vi "CAEN SY5527.vi"() -> ()   [LabVIEW 2018]
uses:
  <vilib>/Instr/_visa.llb/VISA Configure Serial Port (Instr).vi
  <vilib>/Analysis/Matrix/Numeric/Conversions/Matrix To Array - RM.vi
  <vilib>/Analysis/Matrix/NI_Matrix.lvlib
  <instrlib>/CAENHVWrapper/CAENHVWrapper.lvlib
panel:
  in  "MEasuring":T1(tab)
  in  "logs_directory_path":path=path "C:/Users/NEOVP/Documents/HV_DATA"
  in  "Tempt-Presure-on-off":bool=TRUE
  in  "Group 2 log name":string="G2"
  in  "Offsets 2":bool
  out "Temperature [C]":dbl
  in  "COM Port":refnum<visa-resource-name>="COM5"
  out "Presure [Pa]":i32
  in  "Delay [s]":dbl=1.0
  in  "Graphs bachground Color":u32(colorbox)=16448250
  in  "IP Address":string="192.168.0.1"
  in  "Username":string="admin"
  in  "Password":string="admin"
  out "crate_map":string[][](table)
  in  "stop":bool
  in  "Group 1 log name":string="G1"
  in  "Offsets":bool
  in  "Pages Colors":u32[](array[colorbox])=[6901059, 10986955, 11240591, 32639, 32639, 32639, 32639, 16777224, 9868950, 4417895, 8686180, 8686180, 8686180, 8686180]
  in  "Group 1":u16(ring)=5 items=["B0--B1", "B0--B2", "B0--B3", "B1--B0", "B1--B2", "B1--B3", "B2--B0", "B2--B1", "B2--B3", "B3--B0", "B3--B1", "B3--B2"]
  in  "Group 2":u16(ring)=1 items=["B0--B1", "B0--B2", "B0--B3", "B1--B0", "B1--B2", "B1--B3", "B2--B0", "B2--B1", "B2--B3", "B3--B0", "B3--B1", "B3--B2"]
  in  "Set configure":bool
  out "S6-2L R_G1":dbl format="%.1e"
  out "S6-2R R_G1":dbl format="%.1e"
  out "S7-2L R_G1":dbl format="%.1e"
  out "S7-2R R_G1":dbl format="%.1e"
  out "S8-2L R_G1":dbl format="%.1e"
  out "S8-2R R_G1":dbl format="%.1e"
  out "E6-2L R_G1":dbl format="%.1e"
  out "E6-2R R_G1":dbl format="%.1e"
  out "E7-2L R_G1":dbl format="%.1e"
  out "E7-2R R_G1":dbl format="%.1e"
  out "E8-2L R_G1":dbl format="%.1e"
  out "E8-2R R_G1":dbl format="%.1e"
  out "E6-1L R_G1":dbl format="%.1e"
  out "E6-1R R_G1":dbl format="%.1e"
  out "E7-1L R_G1":dbl format="%.1e"
  out "E7-1R R_G1":dbl format="%.1e"
  out "E8-1L R_G1":dbl format="%.1e"
  out "E8-1R R_G1":dbl format="%.1e"
  out "S6-1L R_G1":dbl format="%.1e"
  out "S6-1R R_G1":dbl format="%.1e"
  out "S7-1L R_G1":dbl format="%.1e"
  out "S7-1R R_G1":dbl format="%.1e"
  out "S8-1L R_G1":dbl format="%.1e"
  out "S8-1R R_G1":dbl format="%.1e"
  out "E8-2R I":dbl format="%.3f"
  out "E8-2R V":dbl format="%.1f"
  out "8-R_Gr_L3":bool
  in  "Limits":cluster{dbl, dbl}(slide)={80.16806722689076, 30.252100840336134} scale=0.0..120.0
  out "E6-1R I":dbl format="%.3f"
  out "E6-1R V":dbl format="%.1f"
  out "E6-1L V":dbl format="%.1f"
  out "E6-1L I":dbl format="%.3f"
  out "E7-1R I":dbl format="%.3f"
  out "E7-1R V":dbl format="%.1f"
  out "E7-1L V":dbl format="%.1f"
  out "E7-1L I":dbl format="%.3f"
  out "E8-1R I":dbl format="%.3f"
  out "E8-1R V":dbl format="%.1f"
  out "E8-1L V":dbl format="%.1f"
  out "E8-1L I":dbl format="%.3f"
  out "E6-2R I":dbl format="%.3f"
  out "E6-2R V":dbl format="%.1f"
  out "E6-2L V":dbl format="%.1f"
  out "E6-2L I":dbl format="%.3f"
  out "E7-2R I":dbl format="%.3f"
  out "E7-2R V":dbl format="%.1f"
  out "E7-2L V":dbl format="%.1f"
  out "E7-2L I":dbl format="%.3f"
  out "E8-2L V":dbl format="%.1f"
  out "E8-2L I":dbl format="%.3f"
  out "S6-1R I":dbl format="%.3f"
  out "S6-1R V":dbl format="%.1f"
  out "S6-1L V":dbl format="%.1f"
  out "S6-1L I":dbl format="%.3f"
  out "S7-1R I":dbl format="%.3f"
  out "S7-1R V":dbl format="%.1f"
  out "S7-1L V":dbl format="%.1f"
  out "S7-1L I":dbl format="%.3f"
  out "S8-1R I":dbl format="%.3f"
  out "S8-1R V":dbl format="%.1f"
  out "S8-1L V":dbl format="%.1f"
  out "S8-1L I":dbl format="%.3f"
  out "S6-2R I":dbl format="%.3f"
  out "S6-2R V":dbl format="%.1f"
  out "S6-2L V":dbl format="%.1f"
  out "S6-2L I":dbl format="%.3f"
  out "S7-2R I":dbl format="%.3f"
  out "S7-2R V":dbl format="%.1f"
  out "S7-2L V":dbl format="%.1f"
  out "S7-2L I":dbl format="%.3f"
  out "S8-2R I":dbl format="%.3f"
  out "S8-2R V":dbl format="%.1f"
  out "S8-2L V":dbl format="%.1f"
  out "S8-2L I":dbl format="%.3f"
  out "6-L_Gr_L4":bool
  out "6-R_Gr_L4":bool
  out "7-L_Gr_L4":bool
  out "7-R_Gr_L4":bool
  out "8-L_Gr_L4":bool
  out "8-R_Gr_L4":bool
  out "6-L_Gr_L3":bool
  out "6-R_Gr_L3":bool
  out "7-L_Gr_L3":bool
  out "7-R_Gr_L3":bool
  out "8-L_Gr_L3":bool
  out "6-L_Gr_L2":bool
  out "6-R_Gr_L2":bool
  out "7-L_Gr_L2":bool
  out "7-R_Gr_L2":bool
  out "8-L_Gr_L2":bool
  out "8-R_Gr_L2":bool
  out "6-L_Gr_L1":bool
  out "6-R_Gr_L1":bool
  out "7-L_Gr_L1":bool
  out "7-R_Gr_L1":bool
  out "8-L_Gr_L1":bool
  out "8-R_Gr_L1":bool
  out "8-R_G_L1":bool
  out "8-L_G_L1":bool
  out "8-L_Y_L1":bool
  out "8-R_Y_L1":bool
  out "8-L_R_L1":bool
  out "6-R_R_L1":bool
  out "6-R_Y_L1":bool
  out "6-R_G_L1":bool
  out "6-L_R_L1":bool
  out "6-L_Y_L1":bool
  out "6-L_G_L1":bool
  out "7-R_G_L1":bool
  out "8-R_R_L1":bool
  out "7-L_R_L1":bool
  out "7-L_G_L1":bool
  out "7-R_R_L1":bool
  out "7-L_Y_L1":bool
  out "7-R_Y_L1":bool
  out "8-R_G_L3":bool
  out "8-L_G_L3":bool
  out "8-L_Y_L3":bool
  out "8-R_Y_L3":bool
  out "8-L_R_L3":bool
  out "6-R_R_L3":bool
  out "6-R_Y_L3":bool
  out "6-R_G_L3":bool
  out "6-L_R_L3":bool
  out "6-L_Y_L3":bool
  out "6-L_G_L3":bool
  out "7-R_G_L3":bool
  out "8-R_R_L3":bool
  out "7-L_R_L3":bool
  out "7-L_G_L3":bool
  out "7-R_R_L3":bool
  out "7-L_Y_L3":bool
  out "7-R_Y_L3":bool
  out "8-R_G_L2":bool
  out "8-L_G_L2":bool
  out "8-L_Y_L2":bool
  out "8-R_Y_L2":bool
  out "8-L_R_L2":bool
  out "6-R_R_L2":bool
  out "6-R_Y_L2":bool
  out "6-R_G_L2":bool
  out "6-L_R_L2":bool
  out "6-L_Y_L2":bool
  out "6-L_G_L2":bool
  out "7-R_G_L2":bool
  out "8-R_R_L2":bool
  out "7-L_R_L2":bool
  out "7-L_G_L2":bool
  out "7-R_R_L2":bool
  out "7-L_Y_L2":bool
  out "7-R_Y_L2":bool
  out "8-R_G_L4":bool
  out "8-L_G_L4":bool
  out "8-L_Y_L4":bool
  out "8-R_Y_L4":bool
  out "8-L_R_L4":bool
  out "6-R_R_L4":bool
  out "6-R_Y_L4":bool
  out "6-R_G_L4":bool
  out "6-L_R_L4":bool
  out "6-L_Y_L4":bool
  out "6-L_G_L4":bool
  out "7-R_G_L4":bool
  out "8-R_R_L4":bool
  out "7-L_R_L4":bool
  out "7-L_G_L4":bool
  out "7-R_R_L4":bool
  out "7-L_Y_L4":bool
  out "7-R_Y_L4":bool
  out "Start Time_Currents_Graphs":string
  out "L1 (St-2)":cluster{timestamp[], dbl[]}[](graph)
  out "L2 (St-1)":cluster{timestamp[], dbl[]}[](graph)
  out "L3 (Eta-2 )":cluster{timestamp[], dbl[]}[](graph)
  out "L4 (Eta-1)":cluster{timestamp[], dbl[]}[](graph)
  in  "Logarithm scale 2":bool
  in  "Full_Clear_5":bool
  out "Start Time_L1":string
  out "L1_S6-2L_ind":i64
  out "L1_S6-2R_ind":i64
  out "L1_S7-2L_ind":i64
  out "L1_S7-2R_ind":i64
  out "L1_S8-2L_ind":i64
  out "L1_S8-2R_ind":i64
  out "L1 (St-2) -I":cluster{timestamp[], dbl[]}[](graph)
  out "L1 (St-2) -V":T2(graph)
  in  "Logarithm scale":bool
  in  "Clear_L1":bool
  in  "Full_Clear_1":bool
  out "Start Time_L2":string
  out "L2_S6-1L_ind":i64
  out "L2_S6-1R_ind":i64
  out "L2_S7-1L_ind":i64
  out "L2_S7-1R_ind":i64
  out "L2_S8-1L_ind":i64
  out "L2_S8-1R_ind":i64
  out "L2 (St-1) -I":cluster{timestamp[], dbl[]}[](graph)
  out "L2 (St-1) -V":T2(graph)
  in  "Logarithm scale 3":bool
  in  "Clear_L2":bool
  in  "Full_Clear_2":bool
  out "Start Time_L3":string
  out "L3_E6-2L_ind":i64
  out "L3_E6-2R_ind":i64
  out "L3_E7-2L_ind":i64
  out "L3_E7-2R_ind":i64
  out "L3_E8-2L_ind":i64
  out "L3_E8-2R_ind":i64
  out "L3 (Eta-2) -I":cluster{timestamp[], dbl[]}[](graph)
  out "L3 (Eta-2) -V":T2(graph)
  in  "Logarithm scale 4":bool
  in  "Full_Clear_3":bool
  in  "Clear_L3":bool
  out "Start Time_L4":string
  out "L4_E6-1L_ind":i64
  out "L4_E6-1R_ind":i64
  out "L4_E7-1L_ind":i64
  out "L4_E7-1R_ind":i64
  out "L4_E8-1L_ind":i64
  out "L4_E8-1R_ind":i64
  out "L4 (Eta-1) -I":cluster{timestamp[], dbl[]}[](graph)
  out "L4 (Eta-1) -V":T2(graph)
  in  "Logarithm scale 5":bool
  in  "Clear_L4":bool
  in  "Full_Clear_4":bool
  out "Start Time_T_P":string
  out "Temperature Graph":cluster{timestamp[], dbl[]}(graph)
  out "Presure Graph":cluster{timestamp[], i32[]}(graph)
  out "S8-2L I 2":dbl format="%.3f"
  out "S8-2L V 2":dbl format="%.1f"
  out "S8-2R V 2":dbl format="%.1f"
  out "S8-2R I 2":dbl format="%.3f"
  out "S7-2L I 2":dbl format="%.3f"
  out "S7-2L V 2":dbl format="%.1f"
  out "S7-2R V 2":dbl format="%.1f"
  out "S7-2R I 2":dbl format="%.3f"
  out "S6-2L I 2":dbl format="%.3f"
  out "S6-2L V 2":dbl format="%.1f"
  out "S6-2R V 2":dbl format="%.1f"
  out "S6-2R I 2":dbl format="%.3f"
  out "S8-1L I 2":dbl format="%.3f"
  out "S8-1L V 2":dbl format="%.1f"
  out "S8-1R V 2":dbl format="%.1f"
  out "S8-1R I 2":dbl format="%.3f"
  out "S7-1L I 2":dbl caption="S7-1L I" format="%.3f"
  out "S7-1L V 2":dbl format="%.1f"
  out "S7-1R V 2":dbl format="%.1f"
  out "S7-1R I 2":dbl format="%.3f"
  out "S6-1L I 2":dbl format="%.3f"
  out "S6-1L V 2":dbl format="%.1f"
  out "S6-1R V 2":dbl format="%.1f"
  out "S6-1R I 2":dbl format="%.3f"
  out "E8-2L I 2":dbl format="%.3f"
  out "E8-2L V 2":dbl format="%.1f"
  out "E7-2L I 2":dbl format="%.3f"
  out "E7-2L V 2":dbl format="%.1f"
  out "E7-2R V 2":dbl format="%.1f"
  out "E7-2R I 2":dbl format="%.3f"
  out "E6-2L I 2":dbl format="%.3f"
  out "E6-2L V 2":dbl format="%.1f"
  out "E6-2R V 2":dbl format="%.1f"
  out "E6-2R I 2":dbl format="%.3f"
  out "E8-1L I 2":dbl format="%.3f"
  out "E8-1L V 2":dbl format="%.1f"
  out "E8-1R V 2":dbl format="%.1f"
  out "E8-1R I 2":dbl format="%.3f"
  out "E7-1L I 2":dbl format="%.3f"
  out "E7-1L V 2":dbl format="%.1f"
  out "E7-1R V 2":dbl format="%.1f"
  out "E7-1R I 2":dbl format="%.3f"
  out "E6-1L I 2":dbl format="%.3f"
  out "E6-1L V 2":dbl format="%.1f"
  out "E6-1R V 2":dbl format="%.1f"
  out "E6-1R I 2":dbl format="%.3f"
  out "E8-2R V 2":dbl format="%.1f"
  out "E8-2R I 2":dbl format="%.3f"
  out "8-R_Gr_L3 2":bool
  in  "Limits 2":cluster{dbl, dbl}(slide)={80.16806722689076, 30.252100840336134} scale=0.0..120.0
  out "6-L_Gr_L4 2":bool
  out "6-R_Gr_L4 2":bool
  out "7-L_Gr_L4 2":bool
  out "7-R_Gr_L4 2":bool
  out "8-L_Gr_L4 2":bool
  out "8-R_Gr_L4 2":bool
  out "6-L_Gr_L3 2":bool
  out "6-R_Gr_L3 2":bool
  out "7-L_Gr_L3 2":bool
  out "7-R_Gr_L3 2":bool
  out "8-L_Gr_L3 2":bool
  out "6-L_Gr_L2 2":bool
  out "6-R_Gr_L2 2":bool
  out "7-L_Gr_L2 2":bool
  out "7-R_Gr_L2 2":bool
  out "8-L_Gr_L2 2":bool
  out "8-R_Gr_L2 2":bool
  out "6-L_Gr_L1 2":bool
  out "6-R_Gr_L1 2":bool
  out "7-L_Gr_L1 2":bool
  out "7-R_Gr_L1 2":bool
  out "8-L_Gr_L1 2":bool
  out "8-R_Gr_L1 2":bool
  out "8-R_G_L1 2":bool
  out "8-L_G_L1 2":bool
  out "8-L_Y_L1 2":bool
  out "8-R_Y_L1 2":bool
  out "8-L_R_L1 2":bool
  out "6-R_R_L1 2":bool
  out "6-R_Y_L1 2":bool
  out "6-R_G_L1 2":bool
  out "6-L_R_L1 2":bool
  out "6-L_Y_L1 2":bool
  out "6-L_G_L1 2":bool
  out "7-R_G_L1 2":bool
  out "8-R_R_L1 2":bool
  out "7-L_R_L1 2":bool
  out "7-L_G_L1 2":bool
  out "7-R_R_L1 2":bool
  out "7-L_Y_L1 2":bool
  out "7-R_Y_L1 2":bool
  out "8-R_G_L3 2":bool
  out "8-L_G_L3 2":bool
  out "8-L_Y_L3 2":bool
  out "8-R_Y_L3 2":bool
  out "8-L_R_L3 2":bool
  out "6-R_R_L3 2":bool
  out "6-R_Y_L3 2":bool
  out "6-R_G_L3 2":bool
  out "6-L_R_L3 2":bool
  out "6-L_Y_L3 2":bool
  out "6-L_G_L3 2":bool
  out "7-R_G_L3 2":bool
  out "8-R_R_L3 2":bool
  out "7-L_R_L3 2":bool
  out "7-L_G_L3 2":bool
  out "7-R_R_L3 2":bool
  out "7-L_Y_L3 2":bool
  out "7-R_Y_L3 2":bool
  out "8-R_G_L2 2":bool
  out "8-L_G_L2 2":bool
  out "8-L_Y_L2 2":bool
  out "8-R_Y_L2 2":bool
  out "8-L_R_L2 2":bool
  out "6-R_R_L2 2":bool
  out "6-R_Y_L2 2":bool
  out "6-R_G_L2 2":bool
  out "6-L_R_L2 2":bool
  out "6-L_Y_L2 2":bool
  out "6-L_G_L2 2":bool
  out "7-R_G_L2 2":bool
  out "8-R_R_L2 2":bool
  out "7-L_R_L2 2":bool
  out "7-L_G_L2 2":bool
  out "7-R_R_L2 2":bool
  out "7-L_Y_L2 2":bool
  out "7-R_Y_L2 2":bool
  out "8-R_G_L4 2":bool
  out "8-L_G_L4 2":bool
  out "8-L_Y_L4 2":bool
  out "8-R_Y_L4 2":bool
  out "8-L_R_L4 2":bool
  out "6-R_R_L4 2":bool
  out "6-R_Y_L4 2":bool
  out "6-R_G_L4 2":bool
  out "6-L_R_L4 2":bool
  out "6-L_Y_L4 2":bool
  out "6-L_G_L4 2":bool
  out "7-R_G_L4 2":bool
  out "8-R_R_L4 2":bool
  out "7-L_R_L4 2":bool
  out "7-L_G_L4 2":bool
  out "7-R_R_L4 2":bool
  out "7-L_Y_L4 2":bool
  out "7-R_Y_L4 2":bool
  out "Start Time_Currents_Graphs 2":string
  in  "Full_Clear_5 2":bool
  in  "Logarithm scale 6":bool
  out "L4 (Eta-1) 2":cluster{timestamp[], dbl[]}[](graph)
  out "L3 (Eta-2 ) 2":cluster{timestamp[], dbl[]}[](graph)
  out "L2 (St-1) 2":cluster{timestamp[], dbl[]}[](graph)
  out "L1 (St-2)  2":cluster{timestamp[], dbl[]}[](graph)
  out "Start Time_L1 2":string
  out "L1_S6-2L_ind 2":i64
  out "L1_S6-2R_ind 2":i64
  out "L1_S7-2L_ind 2":i64
  out "L1_S7-2R_ind 2":i64
  out "L1_S8-2L_ind 2":i64
  out "L1_S8-2R_ind 2":i64
  out "L1 (St-2) -I 2":cluster{timestamp[], dbl[]}[](graph)
  out "L1 (St-2) -V 2":T2(graph) caption="L1 (St-2) -V"
  in  "Logarithm scale 7":bool
  in  "Clear_L1 2":bool
  in  "Full_Clear_1 2":bool
  out "Start Time_L2 2":string
  out "L2_S6-1L_ind 2":i64
  out "L2_S6-1R_ind 2":i64
  out "L2_S7-1L_ind 2":i64
  out "L2_S7-1R_ind 2":i64
  out "L2_S8-1L_ind 2":i64
  out "L2_S8-1R_ind 2":i64
  out "L2 (St-1) -I 2":cluster{timestamp[], dbl[]}[](graph)
  out "L2 (St-1) -V 2":T2(graph)
  in  "Logarithm scale 8":bool
  in  "Clear_L2 2":bool
  in  "Full_Clear_2 2":bool
  out "Start Time_L3 2":string
  out "L3_E6-2L_ind 2":i64
  out "L3_E6-2R_ind 2":i64
  out "L3_E7-2L_ind 2":i64
  out "L3_E7-2R_ind 2":i64
  out "L3_E8-2L_ind 2":i64
  out "L3_E8-2R_ind 2":i64
  out "L3 (Eta-2) -I 2":cluster{timestamp[], dbl[]}[](graph)
  out "L3 (Eta-2) -V 2":T2(graph)
  in  "Logarithm scale 9":bool
  in  "Full_Clear_3 2":bool
  in  "Clear_L3 2":bool
  out "Start Time_L4 2":string
  out "L4_E6-1L_ind 2":i64
  out "L4_E6-1R_ind 2":i64
  out "L4_E7-1L_ind 2":i64
  out "L4_E7-1R_ind 2":i64
  out "L4_E8-1L_ind 2":i64
  out "L4_E8-1R_ind 2":i64
  out "L4 (Eta-1) -I 2":cluster{timestamp[], dbl[]}[](graph)
  out "L4 (Eta-1) -V 2":T2(graph)
  in  "Logarithm scale 10":bool
  in  "Clear_L4 2":bool
  in  "Full_Clear_4 2":bool
  # "HV Power Supply Configuration"
  # "Data Save Configuration"
  # "Path of Directory"
  # "Temperature-Presure Configuration"
  # "Ofsets"
  # "Boards grouping"
  # "Graphs bachground Color"
  # "Pages Color"
  # "L1 (St-2)"
  # "L3 (Eta-2)"
  # "E8-2L"
  # "E8-2R"
  # "S8-2L"
  # "13"
  # "S8-2R"
  # "1"
  # "14"
  # "2"
  # "I"
  # "V"
  # "V"
  # "I"
  # "I"
  # "V"
  # "V"
  # "I"
  # "E7-2L"
  # "E7-2R"
  # "S7-2L"
  # "S7-2R"
  # "15"
  # "3"
  # "16"
  # "4"
  # "I"
  # "V"
  # "V"
  # "I"
  # "I"
  # "V"
  # "V"
  # "I"
  # "E6-2L"
  # "E6-2R"
  # "S6-2L"
  # "S6-2R"
  # "17"
  # "5"
  # "18"
  # "6"
  # "I"
  # "V"
  # "V"
  # "I"
  # "I"
  # "V"
  # "V"
  # "I"
  # "Limits"
  # "nA"
  # "L2 (St-1)"
  # "L4 (Eta-1)"
  # "S8-1L"
  # "S8-1R"
  # "E8-1L"
  # "E8-1R"
  # "19"
  # "8"
  # "7"
  # "20"
  # "I"
  # "V"
  # "V"
  # "I"
  # "I"
  # "V"
  # "V"
  # "I"
  # "S7-1L"
  # "S7-1R"
  # "E7-1L"
  # "E7-1R"
  # "9"
  # "21"
  # "10"
  # "22"
  # "I"
  # "V"
  # "V"
  # "I"
  # "I"
  # "V"
  # "V"
  # "I"
  # "S6-1L"
  # "S6-1R"
  # "E6-1L"
  # "E6-1R"
  # "11"
  # "23"
  # "12"
  # "24"
  # "I"
  # "V"
  # "V"
  # "I"
  # "I"
  # "V"
  # "V"
  # "I"
  # "V"
  # "V"
  # "V"
  # "V"
  # "V"
  # "V"
  # "V"
  # "V"
  # "V"
  # "V"
  # "V"
  # "V"
  # "V"
  # "V"
  # "V"
  # "V"
  # "V"
  # "V"
  # "V"
  # "V"
  # "V"
  # "V"
  # "V"
  # "V"
  # "L1 (St-2)"
  # "L3 (Eta-2)"
  # "E8-2L"
  # "E8-2R"
  # "S8-2L"
  # "13"
  # "S8-2R"
  # "1"
  # "14"
  # "2"
  # "I"
  # "V"
  # "V"
  # "I"
  # "I"
  # "V"
  # "V"
  # "I"
  # "E7-2L"
  # "E7-2R"
  # "S7-2L"
  # "S7-2R"
  # "15"
  # "3"
  # "16"
  # "4"
  # "I"
  # "V"
  # "V"
  # "I"
  # "I"
  # "V"
  # "V"
  # "I"
  # "E6-2L"
  # "E6-2R"
  # "S6-2L"
  # "S6-2R"
  # "17"
  # "5"
  # "18"
  # "6"
  # "I"
  # "V"
  # "V"
  # "I"
  # "I"
  # "V"
  # "V"
  # "I"
  # "Limits"
  # "nA"
  # "L2 (St-1)"
  # "L4 (Eta-1)"
  # "S8-1L"
  # "S8-1R"
  # "E8-1L"
  # "E8-1R"
  # "19"
  # "8"
  # "7"
  # "20"
  # "I"
  # "V"
  # "V"
  # "I"
  # "I"
  # "V"
  # "V"
  # "I"
  # "S7-1L"
  # "S7-1R"
  # "E7-1L"
  # "E7-1R"
  # "9"
  # "21"
  # "10"
  # "22"
  # "I"
  # "V"
  # "V"
  # "I"
  # "I"
  # "V"
  # "V"
  # "I"
  # "S6-1L"
  # "S6-1R"
  # "E6-1L"
  # "E6-1R"
  # "11"
  # "23"
  # "12"
  # "24"
  # "I"
  # "V"
  # "V"
  # "I"
  # "I"
  # "V"
  # "V"
  # "I"
  # "V"
  # "V"
  # "V"
  # "V"
  # "V"
  # "V"
  # "V"
  # "V"
  # "V"
  # "V"
  # "V"
  # "V"
  # "V"
  # "V"
  # "V"
  # "V"
  # "V"
  # "V"
  # "V"
  # "V"
  # "V"
  # "V"
  # "V"
  # "V"
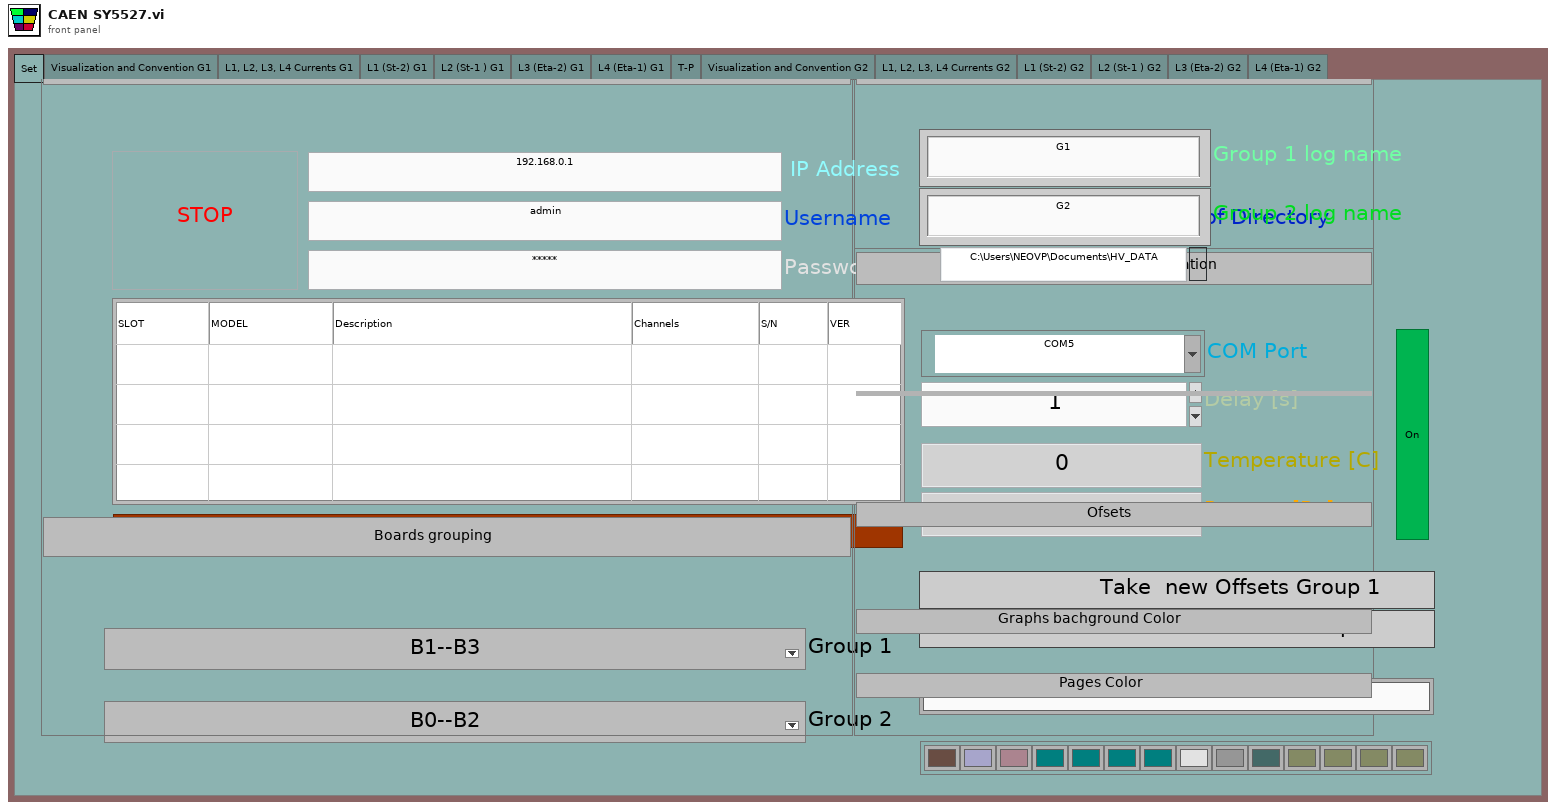
[diagram p1: front panel]
types:
  T1 = enum32{"Set", "Visualization and Convention G1", "L1, L2, L3, L4 Currents G1", "L1 (St-2) G1", "L2 (St-1 ) G1", "L3 (Eta-2) G1", "L4 (Eta-1) G1", "T-P", "Visualization and Convention G2", "L1, L2, L3, L4 Currents G2", "L1 (St-2) G2", "L2 (St-1 ) G2", "L3 (Eta-2) G2", "L4 (Eta-1) G2"}
  T2 = cluster{"appended array":timestamp[], "Ch 11":dbl[]}[]
  T3 = cluster{"IP":string, "UserName":string, "Password":string, "boards_selector_group 1":i32, "boards_selector_group 2":i32, "log_name_group1":string, "log_name_group2":string, "Port":refnum<visa-resource-name>, "Delay[s]":dbl, "on/off":bool, "Graphs_color":i32, "Pages_color":i64[], "logs_Path":path}
  T4 = typedef "LVDateTimeRec.ctl" = cluster{"fractional second":dbl, "second":i32, "minute":i32, "hour":i32, "day of month":i32, "month":i32, "year":i32, "day of week":i32, "day of year":i32, "DST":i32}
  T5 = cluster{dbl, i32, i32, i32, "day of month":i32, "month":i32, "year":i32, "day of week":i32, "day of year":i32, "DST":i32}
  T6 = cluster{"fractional second":dbl, i32, i32, i32, "day of month":i32, "month":i32, "year":i32, "day of week":i32, "day of year":i32, "DST":i32}
  T7 = typedef "NI_Matrix.lvlib/RealMatrix.ctl" = dbl[][]
  T8 = cluster{"Value":string, "Value":string, "Value":string, "Value":u16, "Value":u16, "Value":string, "Value":string, "Value":refnum<visa-resource-name>, "Value":dbl, "Value":bool, "Value":u32, "Value":u32[], "Value":path}
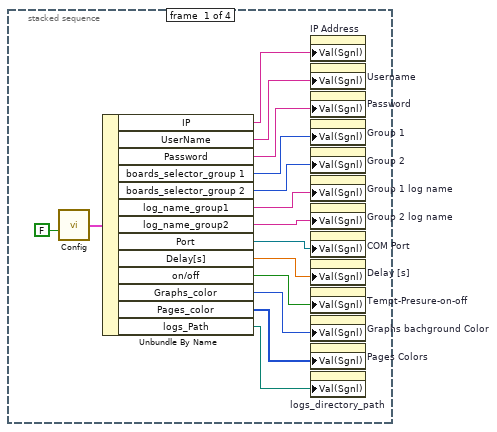
[diagram p2: hidden frame]
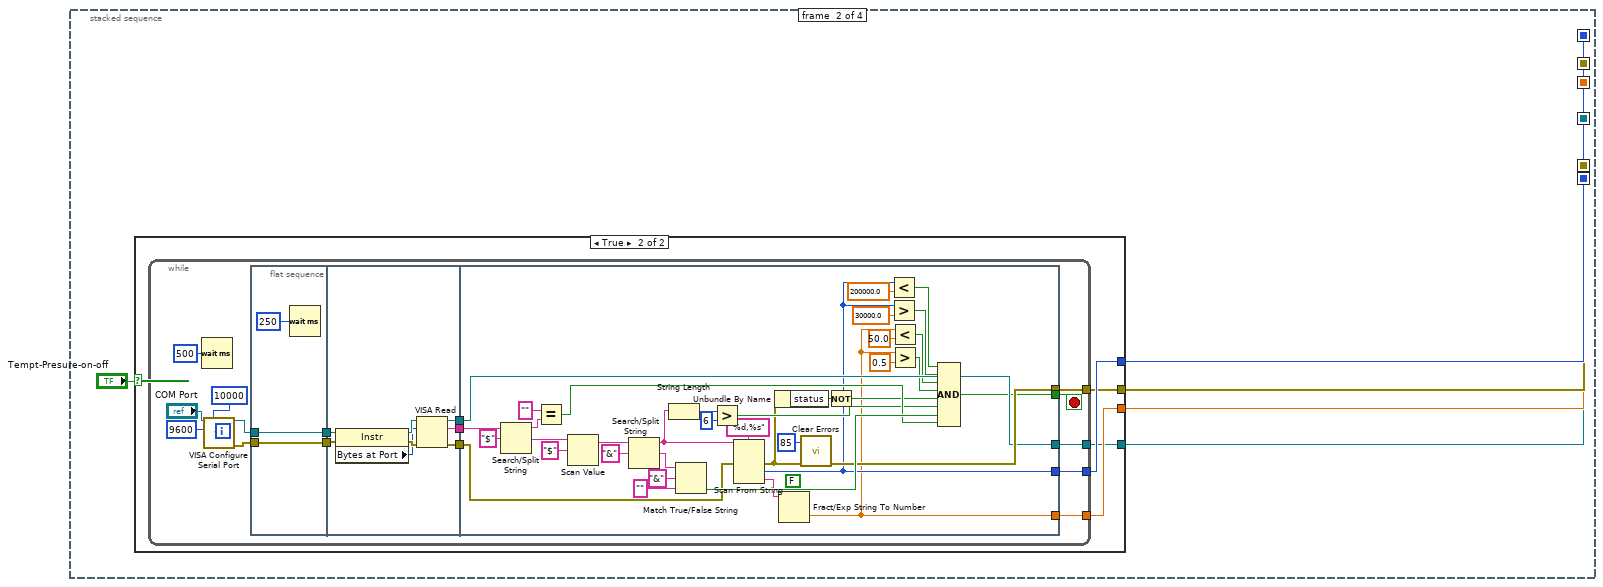
[diagram p3: hidden frame]
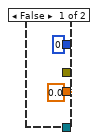
[diagram p4: hidden frame]
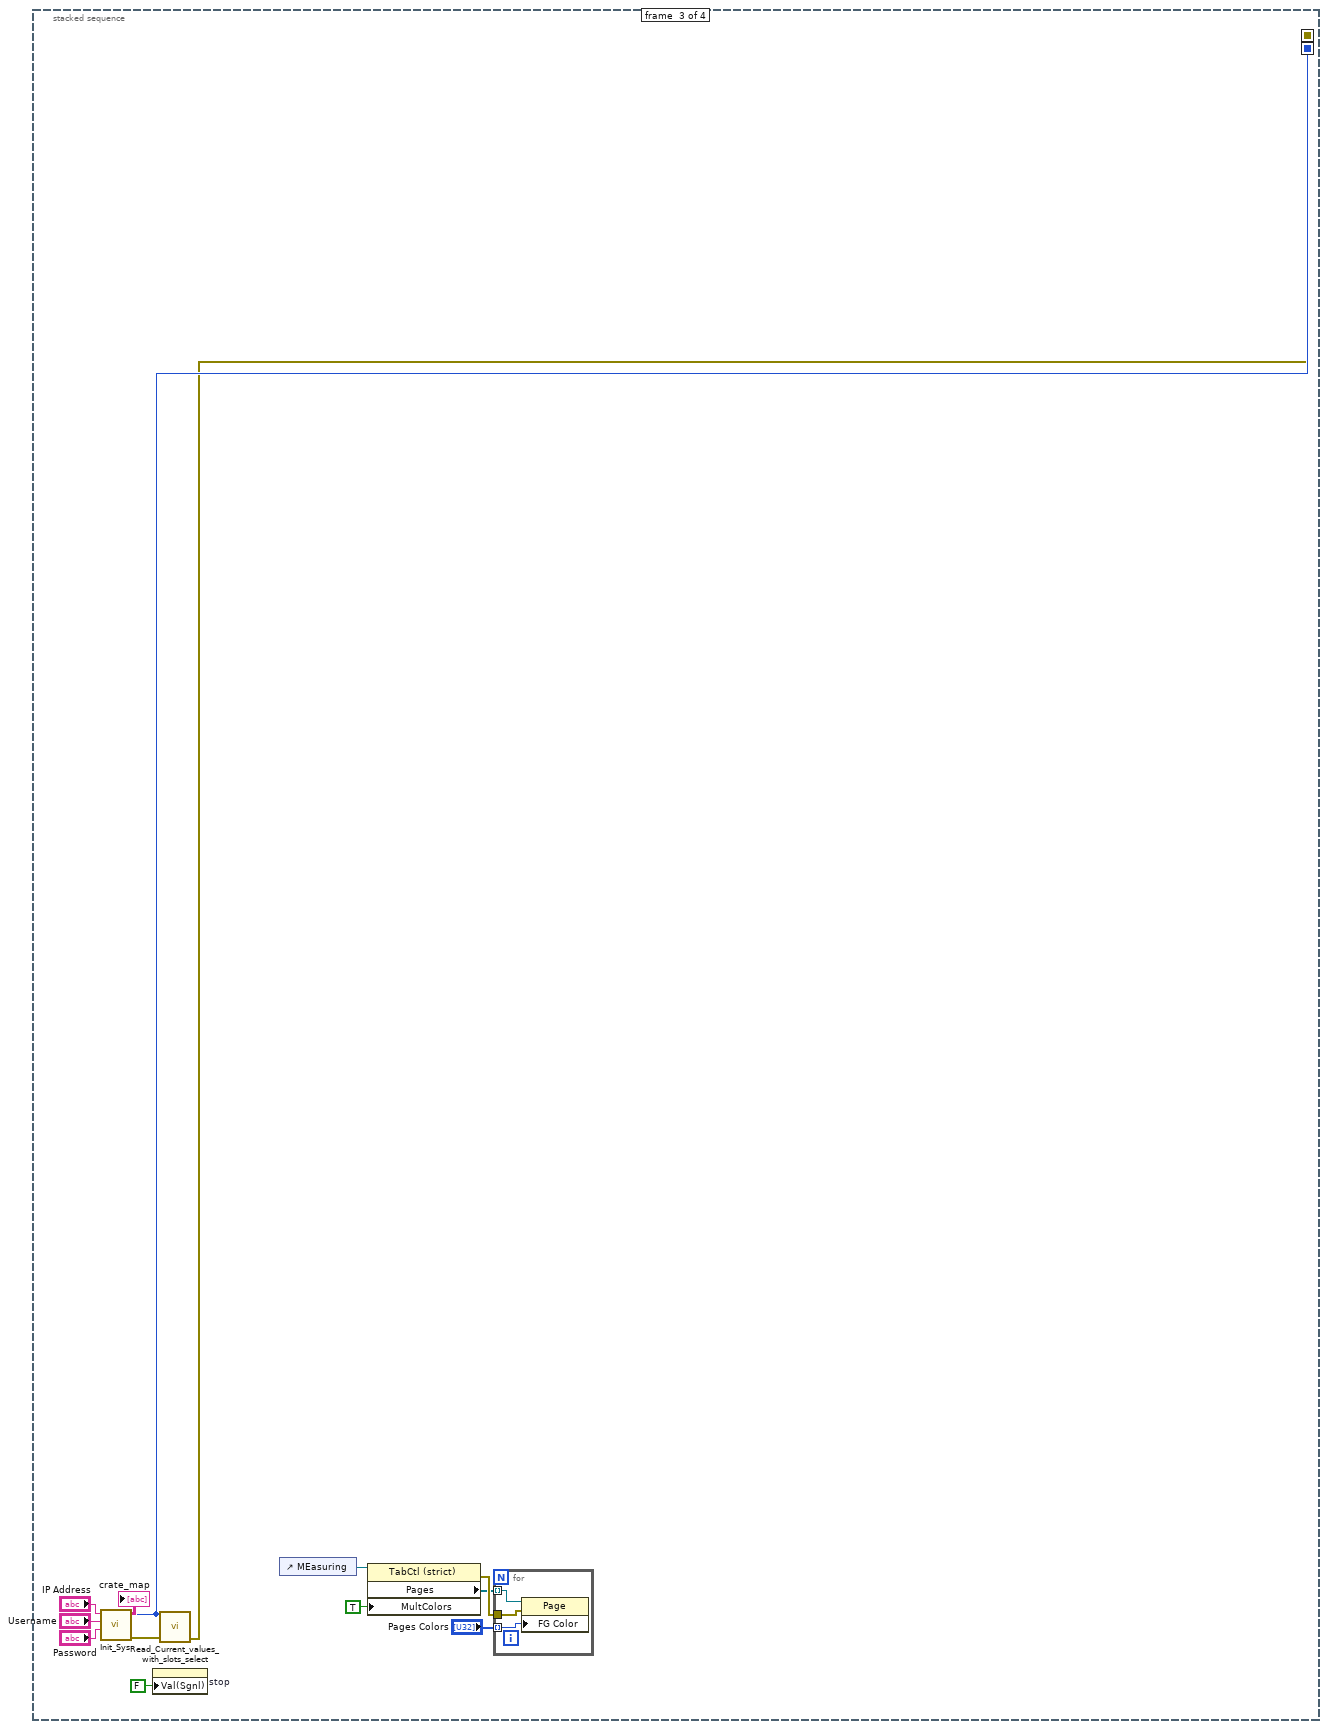
[diagram p5: hidden frame]
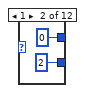
[diagram p6: hidden frame]
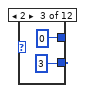
[diagram p7: hidden frame]
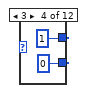
[diagram p8: hidden frame]
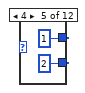
[diagram p9: hidden frame]
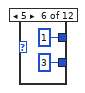
[diagram p10: hidden frame]
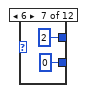
[diagram p11: hidden frame]
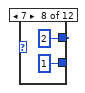
[diagram p12: hidden frame]
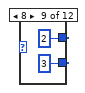
[diagram p13: hidden frame]
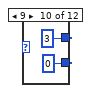
[diagram p14: hidden frame]
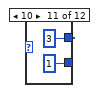
[diagram p15: hidden frame]
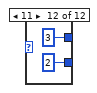
[diagram p16: hidden frame]
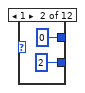
[diagram p17: hidden frame]
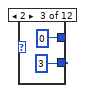
[diagram p18: hidden frame]
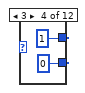
[diagram p19: hidden frame]
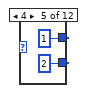
[diagram p20: hidden frame]
diagram:
  n1 = stacked-sequence {
    seq-local: [_ _ w99 _] -> [_ _ _ w123]
    seq-local: [_ _ w97 _] -> [_ _ _ w158]
    seq-local: [_ w16 _ _] -> [_ _ _ w154]
    seq-local: [_ w17 _ _] -> [_ _ _ w156]
    seq-local: [_ w18 _ _] -> [_ _ _ w155]
    seq-local: [_ w19 _ _] -> [_ _ _ w157]
    frame #0 {
      n2 = call "Config.vi"("Config_W/R"=FALSE) -> ("Config_read"=w15:T3)  [unwired: 1 in]
      n3 = Unbundle By Name(w15) -> ("IP"=w14:string, "UserName"=w13:string, "Password"=w12:string, "boards_selector_group 1"=w11:i32, "boards_selector_group 2"=w10:i32, "log_name_group1"=w9:string, "log_name_group2"=w8:string, "Port"=w6:refnum<visa-resource-name>, "Delay[s]"=w5:dbl, "on/off"=w4:bool, "Graphs_color"=w3:i32, "Pages_color"=w2:i64[], "logs_Path"=w1:path)
      n4 = property on="IP Address" class="Str"("Val(Sgnl)"=w14) -> ()  [unwired: 2 in, 2 out]
      n5 = property on="Username" class="Str"("Val(Sgnl)"=w13) -> ()  [unwired: 2 in, 2 out]
      n6 = property on="Password" class="Str"("Val(Sgnl)"=w12) -> ()  [unwired: 2 in, 2 out]
      n7 = property on="Group 1" class="Ring (strict)"("Val(Sgnl)"=w11) -> ()  [unwired: 2 in, 2 out]
      n8 = property on="Group 2" class="Ring (strict)"("Val(Sgnl)"=w10) -> ()  [unwired: 2 in, 2 out]
      n9 = property on="Group 1 log name" class="Str"("Val(Sgnl)"=w9) -> ()  [unwired: 2 in, 2 out]
      n10 = property on="Group 2 log name" class="Str"("Val(Sgnl)"=w8) -> ()  [unwired: 2 in, 2 out]
      n11 = property on="COM Port" class="VISAName"("Val(Sgnl)"=w6) -> ()  [unwired: 2 in, 2 out]
      n12 = property on="Delay [s]" class="DigNum (strict)"("Val(Sgnl)"=w5) -> ()  [unwired: 2 in, 2 out]
      n13 = property on="Tempt-Presure-on-off" class="Bool (strict)"("Val(Sgnl)"=w4) -> ()  [unwired: 2 in, 2 out]
      n14 = property on="Graphs bachground Color" class="ColBox"("Val(Sgnl)"=w3) -> ()  [unwired: 2 in, 2 out]
      n15 = property on="Pages Colors" class="Arr (strict)"("Val(Sgnl)"=w2) -> ()  [unwired: 2 in, 2 out]
      n16 = property on="logs_directory_path" class="Path"("Val(Sgnl)"=w1) -> ()  [unwired: 2 in, 2 out]
    }
    frame #1 {
      n17 = case shown="True" "Tempt-Presure-on-off" {
        tunnel: [0 w26] -> w19
        tunnel: [_ w25] -> w18
        tunnel: [0.0 w24] -> w17
        tunnel: [_ w23] -> w16
        frame False {
        }
        frame True {
          n18 = while {
            tunnel: [w32] -> w25
            tunnel: [w30] -> w26
            tunnel: [w38] -> w24
            tunnel: [w42] -> w23
            stop <- w31 stop-if-true
            n19 = Wait (ms)(milliseconds to wait=u32 500) -> ()  [unwired: 1 out]
            n20 = call-poly "VISA Configure Serial Port"("VISA resource name"="COM Port", "timeout (10sec)"=u32 10000, "baud rate (9600)"=u32 9600) -> ("VISA resource name out"=w33:refnum<visa-resource-name>, "error out"=w34:errorcluster)  [unwired: 11 in]
            n21 = flat-sequence {
              tunnel: w34 -> [w44]
              tunnel: w33 -> [w45]
              tunnel: [w45] -> w28
              tunnel: [w44] -> w27
              tunnel: [w53] -> w41
              tunnel: [w52] -> w40
              tunnel: [w51] -> w39
              tunnel: w28 -> [w50]
              tunnel: w27 -> [w49]
              tunnel: [w65] -> w42
              tunnel: w41 -> [w68]
              tunnel: w40 -> [w65]
              tunnel: w39 -> [w67]
              tunnel: [w58] -> w38
              tunnel: [w66] -> w32
              tunnel: [w64] -> w31
              tunnel: [w59] -> w30
              frame #0 {
                n22 = Wait (ms)(milliseconds to wait=u32 250) -> ()  [unwired: 1 out]
              }
              frame #1 {
                n23 = property class="Instr"(reference=w50, error in=w49) -> (reference out=w48:refnum<visa-resource-name>, error out=w47:errorcluster, "Bytes at Port"=w46:u32)
                n24 = VISA Read(VISA resource name=w48, byte count=w46, error in (no error)=w47) -> (VISA resource name out=w52:refnum<visa-resource-name>, read buffer=w53:string, error out=w51:errorcluster)  [unwired: 1 out]
              }
              frame #2 {
                n25 = Search/Split String(string=w68, search string/char (-)="$") -> (substring before match=w85:string, match + rest of string=w83:string)  [unwired: 1 in, 1 out]
                n26 = Equal?(x="", y=w85) -> (x = y?=w90:bool)
                n27 = Scan Value(string=w83, format string="$") -> (output string=w84:string)  [unwired: 1 in, 1 out]
                n28 = Search/Split String(string=w84, search string/char (-)="&") -> (substring before match=w82:string, match + rest of string=w87:string)  [unwired: 1 in, 1 out]
                n29 = String Length(string=w82) -> (length=w81:i32)
                n30 = Match True/False String(2:"" ("false string"), 3:"&" ("true string"), 4:w87) -> (0:w91:bool)  [unwired: 1 out]
                n31 = Greater?(x=w81, y=6) -> (0:w89:bool)
                n32 = Scan From String(format string="%d,%s", input string=w82, error in=w67) -> (error out=w80:errorcluster, output 1=w59:i32, output 2=w86:string)  [unwired: 3 in, 2 out]
                n33 = Unbundle By Name(w80) -> ("status"=w79:bool)
                n34 = Fract/Exp String To Number(use system decimal point (T)=FALSE, string=w86) -> (number=w58:dbl)  [unwired: 2 in, 1 out]
                n35 = call <vilib>:"Clear Errors.vi"("error in (no error)"=w80, "specific error code to clear (0: all)"=85) -> ("error out"=w66:errorcluster)  [unwired: 4 in, 1 out]
                n36 = Not(x=w79) -> (.not. x?=w88:bool)
                n37 = Less?(x=w59, y=200000.0) -> (x < y?=w54:bool)
                n38 = Greater?(x=w59, y=30000.0) -> (0:w55:bool)
                n39 = Less?(x=w58, y=50.0) -> (x < y?=w56:bool)
                n40 = Greater?(x=w58, y=0.5) -> (0:w57:bool)
                n41 = Compound Arithmetic op=AND(w54, w55, w56, w57, w88, w89, w90, w91) -> (w64:bool)
              }
            }
          }
        }
      }
    }
    frame #2 {
      n42 = call "Init_Sys.vi"("Password"="Password", "Username"="Username", "IP Address"="IP Address") -> ("error out"=w98:errorcluster, "handle"=w99:i32, "crate_map"=→"crate_map":string[][])  [unwired: 6 in]
      n43 = property on="stop" class="Bool"("Val(Sgnl)"=FALSE ("Value (Signaling)")) -> ()  [unwired: 2 in, 2 out]
      n44 = call "Read_Current_values_with_slots_select.vi"("error in"=w98, "handle"=w99) -> ("error out"=w97:errorcluster)  [unwired: 1 in, 5 out]
      n45 = control-ref of="MEasuring"() -> (w96:refnum<vi>)
      n46 = property class="TabCtl (strict)"(reference=w96, "MultColors"=TRUE ("Allow Multiple Colors")) -> (error out=w95:errorcluster, "Pages"=w94:refnum<vi>[])  [unwired: 1 in, 1 out]
      n47 = for {
        tunnel: w95 -> [w106]
        tunnel: "Pages Colors" -> [w105] mode=indexing
        tunnel: w94 -> [w107] mode=indexing
        n48 = property class="Page"(reference=w107, error in=w106, "FG Color"=w105) -> ()  [unwired: 2 out]
      }
    }
    frame #3 {
      w116 = TRUE ("Save")
      w117 = TRUE ("Save 2")
      w121 = sgl[] []
      w122 = sgl[] []
      # "Log file name forming G2"
      # "Log file name forming G1"
      # "Time stamp to sting"
      n49 = Get Date/Time In Seconds() -> (seconds since 1Jan1904=w127:timestamp)
      n50 = Seconds To Date/Time(time stamp (now)=w127) -> (date time rec=w132:T4)  [unwired: 1 in]
      n51 = Seconds To Date/Time(time stamp (now)=w127) -> (date time rec=w150:T4)  [unwired: 1 in]
      n52 = Unbundle By Name(w132) -> ("fractional second"=w135:dbl, "second"=w126:i32, "minute"=w125:i32, "hour"=w124:i32)  [unwired: 6 out]
      n53 = Unbundle By Name(w150) -> ("fractional second"=w149:dbl, "second"=w148:i32, "minute"=w147:i32, "hour"=w146:i32, "day of month"=w134:i32, "month"=w133:i32, "year"=w141:i32, "day of week"=w140:i32, "day of year"=w139:i32, "DST"=w138:i32)
      n54 = Format Date/Time String(seconds (now)=w127) -> (date/time string=w128:string)  [unwired: 2 in]
      n55 = Subtract(x=w135, y=w149) -> (x-y=w145:dbl)
      n56 = call <vilib>:"Search and Replace Pattern.vi"("string"=w128, "regular expression (\"\")"=":" ("regular expression (\"\")"), "replace string (\"\")"="-" ("replace string (\"\")"), "replace all? (F)"=TRUE) -> ("result string"=w110:string)  [unwired: 1 in, 1 out]
      n57 = property on="Start Time_Currents_Graphs" class="Str"("Val(Sgnl)"=w110) -> ()  [unwired: 2 in, 2 out]
      n58 = property on="Start Time_L1" class="Str"("Val(Sgnl)"=w110) -> ()  [unwired: 2 in, 2 out]
      n59 = property on="Start Time_L2" class="Str"("Val(Sgnl)"=w110) -> ()  [unwired: 2 in, 2 out]
      n60 = property on="Start Time_L3" class="Str"("Val(Sgnl)"=w110) -> ()  [unwired: 2 in, 2 out]
      n61 = property on="Start Time_L4" class="Str"("Val(Sgnl)"=w110) -> ()  [unwired: 2 in, 2 out]
      n62 = property on="Start Time_T_P" class="Str"("Val(Sgnl)"=w110) -> ()  [unwired: 2 in, 2 out]
      n63 = property on="Start Time_Currents_Graphs 2" class="Str"("Val(Sgnl)"=w110) -> ()  [unwired: 2 in, 2 out]
      n64 = property on="Start Time_L1 2" class="Str"("Val(Sgnl)"=w110) -> ()  [unwired: 2 in, 2 out]
      n65 = property on="Start Time_L2 2" class="Str"("Val(Sgnl)"=w110) -> ()  [unwired: 2 in, 2 out]
      n66 = property on="Start Time_L3 2" class="Str"("Val(Sgnl)"=w110) -> ()  [unwired: 2 in, 2 out]
      n67 = property on="Start Time_L4 2" class="Str"("Val(Sgnl)"=w110) -> ()  [unwired: 2 in, 2 out]
      n68 = Subtract(x=w126, y=w148) -> (x-y=w144:i32)
      n69 = Subtract(x=w125, y=w147) -> (x-y=w143:i32)
      n70 = local read "logs_directory_path"() -> (w108:path)
      n71 = Subtract(x=w124, y=w146) -> (x-y=w142:i32)
      n72 = Bundle(w145, w144, w143, w142, "day of month"=w134, "month"=w133, "year"=w141, "day of week"=w140, "day of year"=w139, "DST"=w138) -> (w136:T5)  [unwired: 1 in]
      n73 = Concatenate Strings("Group 1 log name", "_" ("string"), w110) -> (w115:string)
      n74 = Concatenate Strings("Group 2 log name", "_" ("string"), w110) -> (w118:string)
      n75 = Date/Time To Seconds(2:w136) -> (0:w137:timestamp)  [unwired: 1 in]
      n76 = Build Array(w127) -> (w161:timestamp[])
      n77 = Build Array(w137) -> (w120:timestamp[])
      n78 = call "Save_Data_file_header_and_path_configuration.vi"("Save"=w117, "path"="logs_directory_path", "File name"=w115) -> ("Output Path"=w151:path)
      n79 = call "Save_Data_file_header_and_path_configuration.vi"("Save"=w116, "path"=w108, "File name"=w118) -> ("Output Path"=w119:path)
      n80 = Build Array(w157) -> (w153:i32[])
      n81 = Build Array(w156) -> (w152:dbl[])
      n82 = while {
        shift-right: [w1346] -> _
        shift-left: w161 -> [w1548]
        shift-right: [w1422] -> _
        shift-left: w122 -> [w1514]
        shift-right: [w1420] -> _
        shift-left: w122 -> [w1513]
        shift-right: [w1418] -> _
        shift-left: w122 -> [w1512]
        shift-right: [w1416] -> _
        shift-left: w122 -> [w1511]
        shift-right: [w1414] -> _
        shift-left: w122 -> [w1510]
        shift-right: [w1412] -> _
        shift-left: w122 -> [w1509]
        shift-right: [w1410] -> _
        shift-left: w122 -> [w1506]
        shift-right: [w1408] -> _
        shift-left: w122 -> [w1505]
        shift-right: [w1406] -> _
        shift-left: w122 -> [w1504]
        shift-right: [w1404] -> _
        shift-left: w122 -> [w1503]
        shift-right: [w1402] -> _
        shift-left: w122 -> [w1502]
        shift-right: [w1400] -> _
        shift-left: w122 -> [w1501]
        shift-right: [w1446] -> _
        shift-left: w122 -> [w1547]
        shift-right: [w1444] -> _
        shift-left: w122 -> [w1546]
        shift-right: [w1442] -> _
        shift-left: w122 -> [w1545]
        shift-right: [w1440] -> _
        shift-left: w122 -> [w1544]
        shift-right: [w1438] -> _
        shift-left: w122 -> [w1543]
        shift-right: [w1436] -> _
        shift-left: w122 -> [w1542]
        shift-right: [w1434] -> _
        shift-left: w122 -> [w1522]
        shift-right: [w1432] -> _
        shift-left: w122 -> [w1521]
        shift-right: [w1430] -> _
        shift-left: w122 -> [w1520]
        shift-right: [w1428] -> _
        shift-left: w122 -> [w1519]
        shift-right: [w1426] -> _
        shift-left: w122 -> [w1518]
        shift-right: [w1424] -> _
        shift-left: w122 -> [w1517]
        tunnel: w117 -> [w1527]
        shift-right: [w1398] -> _
        shift-left: w122 -> [w1496]
        shift-right: [w1396] -> _
        shift-left: w122 -> [w1495]
        shift-right: [w1394] -> _
        shift-left: w122 -> [w1494]
        shift-right: [w1392] -> _
        shift-left: w122 -> [w1493]
        shift-right: [w1390] -> _
        shift-left: w122 -> [w1492]
        shift-right: [w1388] -> _
        shift-left: w122 -> [w1491]
        shift-right: [w1386] -> _
        shift-left: w122 -> [w1490]
        shift-right: [w1384] -> _
        shift-left: w122 -> [w1489]
        shift-right: [w1382] -> _
        shift-left: w122 -> [w1488]
        shift-right: [w1380] -> _
        shift-left: w122 -> [w1487]
        shift-right: [w1378] -> _
        shift-left: w122 -> [w1486]
        shift-right: [w1376] -> _
        shift-left: w122 -> [w1485]
        shift-right: [w1374] -> _
        shift-left: w122 -> [w1484]
        shift-right: [w1372] -> _
        shift-left: w122 -> [w1483]
        shift-right: [w1370] -> _
        shift-left: w122 -> [w1482]
        shift-right: [w1368] -> _
        shift-left: w122 -> [w1481]
        shift-right: [w1366] -> _
        shift-left: w122 -> [w1480]
        shift-right: [w1364] -> _
        shift-left: w122 -> [w1479]
        shift-right: [w1362] -> _
        shift-left: w122 -> [w1478]
        shift-right: [w1360] -> _
        shift-left: w122 -> [w1477]
        shift-right: [w1358] -> _
        shift-left: w122 -> [w1476]
        shift-right: [w1356] -> _
        shift-left: w122 -> [w1475]
        shift-right: [w1354] -> _
        shift-left: w122 -> [w1474]
        shift-right: [w1352] -> _
        shift-left: w122 -> [w1473]
        tunnel: w151 -> [w1528]
        tunnel: w123 -> [w1448]
        tunnel: w158 -> [w1529]
        shift-right: [w1350] -> _
        shift-left: w153 -> [w1287]
        shift-right: [w1348] -> _
        shift-left: w152 -> [w1286]
        tunnel: [w1449] -> w160
        tunnel: [w1448] -> w159
        tunnel: w155 -> [w1284]
        tunnel: w154 -> [w1285]
        tunnel: w153 -> [w1289]
        tunnel: w152 -> [w1288]
        shift-right: [w1229] -> _
        shift-left: w122 -> [w1220]
        shift-right: [w1227] -> _
        shift-left: w122 -> [w1219]
        shift-right: [w1225] -> _
        shift-left: w122 -> [w1218]
        shift-right: [w1223] -> _
        shift-left: w122 -> [w1217]
        shift-right: [w1221] -> _
        shift-left: w122 -> [w1216]
        shift-right: [w1214] -> _
        shift-left: w122 -> [w1213]
        shift-right: [w1209] -> _
        shift-left: w122 -> [w1198]
        shift-right: [w1207] -> _
        shift-left: w122 -> [w1197]
        shift-right: [w1205] -> _
        shift-left: w122 -> [w1196]
        shift-right: [w1203] -> _
        shift-left: w122 -> [w1195]
        shift-right: [w1201] -> _
        shift-left: w122 -> [w1194]
        shift-right: [w1199] -> _
        shift-left: w122 -> [w1193]
        shift-right: [w1190] -> _
        shift-left: w122 -> [w1177]
        shift-right: [w1189] -> _
        shift-left: w122 -> [w1176]
        shift-right: [w1186] -> _
        shift-left: w122 -> [w1175]
        shift-right: [w1184] -> _
        shift-left: w122 -> [w1174]
        shift-right: [w1182] -> _
        shift-left: w122 -> [w1173]
        shift-right: [w1180] -> _
        shift-left: w122 -> [w1172]
        shift-right: [w1178] -> _
        shift-left: w122 -> [w1160]
        shift-right: [w1169] -> _
        shift-left: w122 -> [w1159]
        shift-right: [w1167] -> _
        shift-left: w122 -> [w1158]
        shift-right: [w1165] -> _
        shift-left: w122 -> [w1157]
        shift-right: [w1163] -> _
        shift-left: w122 -> [w1156]
        shift-right: [w1161] -> _
        shift-left: w122 -> [w1155]
        shift-right: [w589] -> _
        shift-left: w120 -> [w1143]
        tunnel: w126 -> [w1127]
        tunnel: w125 -> [w1126]
        tunnel: w124 -> [w1125]
        tunnel: w122 -> [w1098]
        shift-right: [w787] -> _
        shift-left: w121 -> [w708]
        shift-right: [w789] -> _
        shift-left: w121 -> [w709]
        shift-right: [w791] -> _
        shift-left: w121 -> [w710]
        shift-right: [w793] -> _
        shift-left: w121 -> [w711]
        shift-right: [w795] -> _
        shift-left: w121 -> [w712]
        shift-right: [w797] -> _
        shift-left: w121 -> [w713]
        shift-right: [w799] -> _
        shift-left: w121 -> [w715]
        shift-right: [w801] -> _
        shift-left: w121 -> [w716]
        shift-right: [w803] -> _
        shift-left: w121 -> [w717]
        shift-right: [w805] -> _
        shift-left: w121 -> [w718]
        shift-right: [w807] -> _
        shift-left: w121 -> [w719]
        shift-right: [w809] -> _
        shift-left: w121 -> [w720]
        shift-right: [w763] -> _
        shift-left: w121 -> [w682]
        shift-right: [w765] -> _
        shift-left: w121 -> [w683]
        shift-right: [w767] -> _
        shift-left: w121 -> [w684]
        shift-right: [w769] -> _
        shift-left: w121 -> [w685]
        shift-right: [w771] -> _
        shift-left: w121 -> [w686]
        shift-right: [w773] -> _
        shift-left: w121 -> [w687]
        shift-right: [w775] -> _
        shift-left: w121 -> [w700]
        shift-right: [w777] -> _
        shift-left: w121 -> [w701]
        shift-right: [w779] -> _
        shift-left: w121 -> [w702]
        shift-right: [w781] -> _
        shift-left: w121 -> [w703]
        shift-right: [w783] -> _
        shift-left: w121 -> [w704]
        shift-right: [w785] -> _
        shift-left: w121 -> [w705]
        shift-right: [w811] -> _
        shift-left: w121 -> [w725]
        shift-right: [w813] -> _
        shift-left: w121 -> [w726]
        shift-right: [w815] -> _
        shift-left: w121 -> [w727]
        shift-right: [w817] -> _
        shift-left: w121 -> [w728]
        shift-right: [w819] -> _
        shift-left: w121 -> [w729]
        shift-right: [w821] -> _
        shift-left: w121 -> [w730]
        shift-right: [w823] -> _
        shift-left: w121 -> [w731]
        shift-right: [w825] -> _
        shift-left: w121 -> [w732]
        shift-right: [w827] -> _
        shift-left: w121 -> [w733]
        shift-right: [w829] -> _
        shift-left: w121 -> [w734]
        shift-right: [w831] -> _
        shift-left: w121 -> [w735]
        shift-right: [w833] -> _
        shift-left: w121 -> [w736]
        shift-right: [w835] -> _
        shift-left: w121 -> [w737]
        shift-right: [w837] -> _
        shift-left: w121 -> [w738]
        shift-right: [w839] -> _
        shift-left: w121 -> [w739]
        shift-right: [w841] -> _
        shift-left: w121 -> [w740]
        shift-right: [w843] -> _
        shift-left: w121 -> [w741]
        shift-right: [w845] -> _
        shift-left: w121 -> [w742]
        shift-right: [w847] -> _
        shift-left: w121 -> [w743]
        shift-right: [w849] -> _
        shift-left: w121 -> [w744]
        shift-right: [w851] -> _
        shift-left: w121 -> [w745]
        shift-right: [w853] -> _
        shift-left: w121 -> [w746]
        shift-right: [w855] -> _
        shift-left: w121 -> [w747]
        shift-right: [w857] -> _
        shift-left: w121 -> [w748]
        shift-right: [w859] -> _
        shift-left: w121 -> [w868]
        shift-right: [w861] -> _
        shift-left: w121 -> [w869]
        shift-right: [w863] -> _
        shift-left: w121 -> [w870]
        shift-right: [w865] -> _
        shift-left: w121 -> [w871]
        shift-right: [w867] -> _
        shift-left: w121 -> [w872]
        shift-right: [w874] -> _
        shift-left: w121 -> [w875]
        shift-right: [w879] -> _
        shift-left: w121 -> [w890]
        shift-right: [w881] -> _
        shift-left: w121 -> [w891]
        shift-right: [w883] -> _
        shift-left: w121 -> [w892]
        shift-right: [w885] -> _
        shift-left: w121 -> [w893]
        shift-right: [w887] -> _
        shift-left: w121 -> [w894]
        shift-right: [w889] -> _
        shift-left: w121 -> [w895]
        shift-right: [w898] -> _
        shift-left: w121 -> [w911]
        shift-right: [w899] -> _
        shift-left: w121 -> [w912]
        shift-right: [w902] -> _
        shift-left: w121 -> [w913]
        shift-right: [w904] -> _
        shift-left: w121 -> [w914]
        shift-right: [w906] -> _
        shift-left: w121 -> [w915]
        shift-right: [w908] -> _
        shift-left: w121 -> [w916]
        shift-right: [w910] -> _
        shift-left: w121 -> [w928]
        shift-right: [w919] -> _
        shift-left: w121 -> [w929]
        shift-right: [w921] -> _
        shift-left: w121 -> [w930]
        shift-right: [w923] -> _
        shift-left: w121 -> [w931]
        shift-right: [w925] -> _
        shift-left: w121 -> [w932]
        shift-right: [w927] -> _
        shift-left: w121 -> [w933]
        tunnel: w121 -> [w946]
        tunnel: w119 -> [w650]
        tunnel: w116 -> [w649]
        stop <- "stop" stop-if-true
        w292 = 1000.0 ("x")
        w446 = 6 ("length")
        w448 = 6 ("length")
        w555 = 1 ("disabled index (col)")
        w549 = 0 ("disabled index (col)")
        w538 = 1 ("disabled index (col)")
        w544 = 0 ("disabled index (col)")
        w527 = 1 ("disabled index (col)")
        w521 = 0 ("disabled index (col)")
        w510 = 1 ("disabled index (col)")
        w516 = 0 ("disabled index (col)")
        w605 = 1 ("disabled index (col)")
        w620 = 1 ("disabled index (col)")
        w633 = 1 ("disabled index (col)")
        w644 = 1 ("disabled index (col)")
        w941 = 12 ("length")
        w752 = 6 ("length")
        w753 = 0 ("index")
        w751 = 6 ("length")
        w750 = 0 ("index")
        w749 = 12 ("length")
        w947 = 1000.0 ("x")
        w1110 = 12 ("length")
        w1295 = 1 ("disabled index (col)")
        w1301 = 0 ("disabled index (col)")
        w1312 = 1 ("disabled index (col)")
        w1306 = 0 ("disabled index (col)")
        w1323 = 1 ("disabled index (col)")
        w1329 = 0 ("disabled index (col)")
        w1340 = 1 ("disabled index (col)")
        w1334 = 0 ("disabled index (col)")
        w1452 = 6 ("length")
        w1454 = 6 ("length")
        w1465 = 6 ("length")
        w1464 = 0 ("index")
        w1466 = 6 ("length")
        w1467 = 0 ("index")
        w1468 = 12 ("length")
        # "Resistance _G1"
        # "Visualization G1"
        # "Voltages_and_Currents_visualization G2"
        # "Vlotage Indicators Group 1"
        # "Graphs timestamps G2"
        # "Linear-logarithm scale G2"
        # "Data storage for G2"
        # "Data storage for G1"
        # "Data reading"
        # "Graphs timestamps G1"
        # "Voltages_and_Currents_visualization G1"
        # "Linear-logarithm scale G1"
        # "Visualization G1"
        # "Graphs Background colors"
        n83 = local read "S8-2R V"() -> (w263:dbl)
        n84 = local read "S7-2R V"() -> (w259:dbl)
        n85 = local read "S6-2R V"() -> (w255:dbl)
        n86 = local read "S8-2L V"() -> (w261:dbl)
        n87 = local read "S7-2L V"() -> (w257:dbl)
        n88 = local read "S6-2L V"() -> (w253:dbl)
        n89 = local read "S8-2R I"() -> (w262:dbl)
        n90 = local read "S7-2R I"() -> (w258:dbl)
        n91 = local read "S6-2R I"() -> (w254:dbl)
        n92 = local read "S8-2L I"() -> (w260:dbl)
        n93 = local read "S7-2L I"() -> (w256:dbl)
        n94 = local read "S6-2L I"() -> (w230:dbl)
        n95 = local read "Tempt-Presure-on-off"() -> (w1115:bool)
        n96 = case shown="True" w1115 {
          tunnel: w1285 -> [_ w1840]
          tunnel: w1284 -> [_ w1839]
          tunnel: [w1835 w1837] -> w1283
          tunnel: [w1836 w1838] -> w1107
          frame False {
            w1835 = 0 ("Presure [Pa]")
            w1836 = 0.0 ("Temperature [C]")
            n97 = local write "Temperature [C]"(w1836) -> ()
            n98 = local write "Presure [Pa]"(w1835) -> ()
          }
          frame True {
            n99 = while {
              tunnel: w1840 -> [w1847]
              tunnel: w1839 -> [w1846]
              tunnel: [w1842] -> w1838
              tunnel: [w1841] -> w1837
              stop <- w1843 stop-if-true
              n100 = flat-sequence {
                tunnel: w1847 -> [w1854]
                tunnel: w1846 -> [w1853]
                tunnel: [w1849] -> w1845
                tunnel: [w1848] -> w1844
                tunnel: w1845 -> [w1866]
                tunnel: w1844 -> [w1867]
                tunnel: [w1865] -> w1843
                tunnel: [w1856] -> w1842
                tunnel: [w1855] -> w1841
                frame #0 {
                  n101 = property class="Instr"(reference=w1854, error in=w1853) -> (reference out=w1852:refnum<visa-resource-name>, error out=w1851:errorcluster, "Bytes at Port"=w1850:u32)
                  n102 = VISA Read(VISA resource name=w1852, byte count=w1850, error in (no error)=w1851) -> (read buffer=w1849:string, error out=w1848:errorcluster)  [unwired: 2 out]
                }
                frame #1 {
                  n103 = Search/Split String(string=w1866, search string/char (-)="$") -> (substring before match=w1884:string, match + rest of string=w1886:string)  [unwired: 1 in, 1 out]
                  n104 = Equal?(x="", y=w1884) -> (x = y?=w1879:bool)
                  n105 = Scan Value(string=w1886, format string="$") -> (output string=w1885:string)  [unwired: 1 in, 1 out]
                  n106 = Search/Split String(string=w1885, search string/char (-)="&") -> (substring before match=w1887:string, match + rest of string=w1882:string)  [unwired: 1 in, 1 out]
                  n107 = String Length(string=w1887) -> (length=w1888:i32)
                  n108 = Match True/False String(2:"" ("false string"), 3:"&" ("true string"), 4:w1882) -> (0:w1878:bool)  [unwired: 1 out]
                  n109 = Greater?(x=w1888, y=6) -> (0:w1880:bool)
                  n110 = Scan From String(format string="%d,%s", input string=w1887, error in=w1867) -> (error out=w1889:errorcluster, output 1=w1855:i32, output 2=w1883:string)  [unwired: 3 in, 2 out]
                  "Presure [Pa]" <- w1855
                  n111 = Unbundle By Name(w1889) -> ("status"=w1890:bool)
                  n112 = Fract/Exp String To Number(use system decimal point (T)=FALSE, string=w1883) -> (number=w1856:dbl)  [unwired: 2 in, 1 out]
                  "Temperature [C]" <- w1856
                  n113 = call <vilib>:"Clear Errors.vi"("error in (no error)"=w1889, "specific error code to clear (0: all)"=85) -> ()  [unwired: 4 in, 2 out]
                  n114 = Not(x=w1890) -> (.not. x?=w1881:bool)
                  n115 = Less?(x=w1855, y=200000.0) -> (x < y?=w1860:bool)
                  n116 = Greater?(x=w1855, y=30000.0) -> (0:w1859:bool)
                  n117 = Less?(x=w1856, y=40.0) -> (x < y?=w1858:bool)
                  n118 = Greater?(x=w1856, y=10.0) -> (0:w1857:bool)
                  n119 = Compound Arithmetic op=AND(w1881, w1880, w1879, w1878, w1860, w1859, w1858, w1857) -> (w1865:bool)
                }
              }
            }
          }
        }
        n120 = event shown="[5] \"Full_Clear_1 2\", \"Full_Clear_2 2\", \"Full_Clear_3 2\", \"Full_Clear_4 2\", \"Full_Clear_5 2\": Value Change" {
          selector: _ -> [_ _ _ _ _ _]
          dyn-events: _ -> [_ _ _ _ _ _]
          timeout: 1 -> [_ _ _ _ _ _]
          event Timeout {
            n121 = event-data() -> ()  [unwired: 1 in, 3 out]
          }
          event "Clear_L1 2": Value Change {
            n122 = event-data() -> ()  [unwired: 1 in, 3 out]
            n123 = Get Date/Time In Seconds() -> (seconds since 1Jan1904=w1599:timestamp)
            n124 = Format Date/Time String(seconds (now)=w1599) -> (date/time string=w1600:string)  [unwired: 2 in]
            n125 = call <vilib>:"Search and Replace Pattern.vi"("string"=w1600, "regular expression (\"\")"=":" ("regular expression (\"\")"), "replace string (\"\")"="-" ("replace string (\"\")"), "replace all? (F)"=TRUE) -> ("result string"=w1597:string)  [unwired: 1 in, 1 out]
            n126 = property on="Start Time_L1 2" class="Str"("Val(Sgnl)"=w1597) -> ()  [unwired: 2 in, 2 out]
          }
          event "Clear_L2 2": Value Change {
            n127 = event-data() -> ()  [unwired: 1 in, 3 out]
            n128 = Get Date/Time In Seconds() -> (seconds since 1Jan1904=w1607:timestamp)
            n129 = Format Date/Time String(seconds (now)=w1607) -> (date/time string=w1608:string)  [unwired: 2 in]
            n130 = call <vilib>:"Search and Replace Pattern.vi"("string"=w1608, "regular expression (\"\")"=":" ("regular expression (\"\")"), "replace string (\"\")"="-" ("replace string (\"\")"), "replace all? (F)"=TRUE) -> ("result string"=w1603:string)  [unwired: 1 in, 1 out]
            n131 = property on="Start Time_L2 2" class="Str"("Val(Sgnl)"=w1603) -> ()  [unwired: 2 in, 2 out]
          }
          event "Clear_L3 2": Value Change {
            n132 = event-data() -> ()  [unwired: 1 in, 3 out]
            n133 = Get Date/Time In Seconds() -> (seconds since 1Jan1904=w1613:timestamp)
            n134 = Format Date/Time String(seconds (now)=w1613) -> (date/time string=w1614:string)  [unwired: 2 in]
            n135 = call <vilib>:"Search and Replace Pattern.vi"("string"=w1614, "regular expression (\"\")"=":" ("regular expression (\"\")"), "replace string (\"\")"="-" ("replace string (\"\")"), "replace all? (F)"=TRUE) -> ("result string"=w1609:string)  [unwired: 1 in, 1 out]
            n136 = property on="Start Time_L3 2" class="Str"("Val(Sgnl)"=w1609) -> ()  [unwired: 2 in, 2 out]
          }
          event "Clear_L4 2": Value Change {
            n137 = event-data() -> ()  [unwired: 1 in, 4 out]
            n138 = Get Date/Time In Seconds() -> (seconds since 1Jan1904=w1620:timestamp)
            n139 = Format Date/Time String(seconds (now)=w1620) -> (date/time string=w1619:string)  [unwired: 2 in]
            n140 = call <vilib>:"Search and Replace Pattern.vi"("string"=w1619, "regular expression (\"\")"=":" ("regular expression (\"\")"), "replace string (\"\")"="-" ("replace string (\"\")"), "replace all? (F)"=TRUE) -> ("result string"=w1615:string)  [unwired: 1 in, 1 out]
            n141 = property on="Start Time_L4 2" class="Str"("Val(Sgnl)"=w1615) -> ()  [unwired: 2 in, 2 out]
          }
          event "Full_Clear_1 2", "Full_Clear_2 2", "Full_Clear_3 2", "Full_Clear_4 2", "Full_Clear_5 2": Value Change {
            n142 = event-data() -> ()  [unwired: 1 in, 4 out]
            n143 = Get Date/Time In Seconds() -> (seconds since 1Jan1904=w1626:timestamp)
            n144 = Format Date/Time String(seconds (now)=w1626) -> (date/time string=w1625:string)  [unwired: 2 in]
            n145 = call <vilib>:"Search and Replace Pattern.vi"("string"=w1625, "regular expression (\"\")"=":" ("regular expression (\"\")"), "replace string (\"\")"="-" ("replace string (\"\")"), "replace all? (F)"=TRUE) -> ("result string"=w1621:string)  [unwired: 1 in, 1 out]
            n146 = property on="Start Time_L1 2" class="Str"("Val(Sgnl)"=w1621) -> ()  [unwired: 2 in, 2 out]
            n147 = property on="Start Time_L2 2" class="Str"("Val(Sgnl)"=w1621) -> ()  [unwired: 2 in, 2 out]
            n148 = property on="Start Time_L3 2" class="Str"("Val(Sgnl)"=w1621) -> ()  [unwired: 2 in, 2 out]
            n149 = property on="Start Time_L4 2" class="Str"("Val(Sgnl)"=w1621) -> ()  [unwired: 2 in, 2 out]
            n150 = property on="Start Time_Currents_Graphs 2" class="Str"("Val(Sgnl)"=w1621) -> ()  [unwired: 2 in, 2 out]
          }
        }
        n151 = Divide(x=w263, y=w262) -> (x/y=w241:dbl)
        n152 = Divide(x=w261, y=w260) -> (x/y=w238:dbl)
        n153 = Divide(x=w259, y=w258) -> (x/y=w235:dbl)
        n154 = Divide(x=w257, y=w256) -> (x/y=w234:dbl)
        n155 = Divide(x=w255, y=w254) -> (x/y=w239:dbl)
        n156 = Divide(x=w253, y=w230) -> ()  [unwired: 1 out]
        n157 = local read "Temperature [C]"() -> (w1525:dbl)
        n158 = event shown="[5] \"Full_Clear_1\", \"Full_Clear_2\", \"Full_Clear_3\", \"Full_Clear_4\", \"Full_Clear_5\": Value Change" {
          selector: _ -> [_ _ _ _ _ _]
          dyn-events: _ -> [_ _ _ _ _ _]
          timeout: 1 -> [_ _ _ _ _ _]
          event Timeout {
            n159 = event-data() -> ()  [unwired: 1 in, 3 out]
          }
          event "Clear_L1": Value Change {
            n160 = event-data() -> ()  [unwired: 1 in, 3 out]
            n161 = Get Date/Time In Seconds() -> (seconds since 1Jan1904=w1807:timestamp)
            n162 = Format Date/Time String(seconds (now)=w1807) -> (date/time string=w1808:string)  [unwired: 2 in]
            n163 = call <vilib>:"Search and Replace Pattern.vi"("string"=w1808, "regular expression (\"\")"=":" ("regular expression (\"\")"), "replace string (\"\")"="-" ("replace string (\"\")"), "replace all? (F)"=TRUE) -> ("result string"=w1805:string)  [unwired: 1 in, 1 out]
            n164 = property on="Start Time_L1" class="Str"("Val(Sgnl)"=w1805) -> ()  [unwired: 2 in, 2 out]
          }
          event "Clear_L2": Value Change {
            n165 = event-data() -> ()  [unwired: 1 in, 3 out]
            n166 = Get Date/Time In Seconds() -> (seconds since 1Jan1904=w1815:timestamp)
            n167 = Format Date/Time String(seconds (now)=w1815) -> (date/time string=w1816:string)  [unwired: 2 in]
            n168 = call <vilib>:"Search and Replace Pattern.vi"("string"=w1816, "regular expression (\"\")"=":" ("regular expression (\"\")"), "replace string (\"\")"="-" ("replace string (\"\")"), "replace all? (F)"=TRUE) -> ("result string"=w1811:string)  [unwired: 1 in, 1 out]
            n169 = property on="Start Time_L2" class="Str"("Val(Sgnl)"=w1811) -> ()  [unwired: 2 in, 2 out]
          }
          event "Clear_L3": Value Change {
            n170 = event-data() -> ()  [unwired: 1 in, 3 out]
            n171 = Get Date/Time In Seconds() -> (seconds since 1Jan1904=w1821:timestamp)
            n172 = Format Date/Time String(seconds (now)=w1821) -> (date/time string=w1822:string)  [unwired: 2 in]
            n173 = call <vilib>:"Search and Replace Pattern.vi"("string"=w1822, "regular expression (\"\")"=":" ("regular expression (\"\")"), "replace string (\"\")"="-" ("replace string (\"\")"), "replace all? (F)"=TRUE) -> ("result string"=w1817:string)  [unwired: 1 in, 1 out]
            n174 = property on="Start Time_L3" class="Str"("Val(Sgnl)"=w1817) -> ()  [unwired: 2 in, 2 out]
          }
          event "Clear_L4": Value Change {
            n175 = event-data() -> ()  [unwired: 1 in, 4 out]
            n176 = Get Date/Time In Seconds() -> (seconds since 1Jan1904=w1828:timestamp)
            n177 = Format Date/Time String(seconds (now)=w1828) -> (date/time string=w1827:string)  [unwired: 2 in]
            n178 = call <vilib>:"Search and Replace Pattern.vi"("string"=w1827, "regular expression (\"\")"=":" ("regular expression (\"\")"), "replace string (\"\")"="-" ("replace string (\"\")"), "replace all? (F)"=TRUE) -> ("result string"=w1823:string)  [unwired: 1 in, 1 out]
            n179 = property on="Start Time_L4" class="Str"("Val(Sgnl)"=w1823) -> ()  [unwired: 2 in, 2 out]
          }
          event "Full_Clear_1", "Full_Clear_2", "Full_Clear_3", "Full_Clear_4", "Full_Clear_5": Value Change {
            n180 = event-data() -> ()  [unwired: 1 in, 4 out]
            n181 = Get Date/Time In Seconds() -> (seconds since 1Jan1904=w1834:timestamp)
            n182 = Format Date/Time String(seconds (now)=w1834) -> (date/time string=w1833:string)  [unwired: 2 in]
            n183 = call <vilib>:"Search and Replace Pattern.vi"("string"=w1833, "regular expression (\"\")"=":" ("regular expression (\"\")"), "replace string (\"\")"="-" ("replace string (\"\")"), "replace all? (F)"=TRUE) -> ("result string"=w1829:string)  [unwired: 1 in, 1 out]
            n184 = property on="Start Time_L1" class="Str"("Val(Sgnl)"=w1829) -> ()  [unwired: 2 in, 2 out]
            n185 = property on="Start Time_L2" class="Str"("Val(Sgnl)"=w1829) -> ()  [unwired: 2 in, 2 out]
            n186 = property on="Start Time_L3" class="Str"("Val(Sgnl)"=w1829) -> ()  [unwired: 2 in, 2 out]
            n187 = property on="Start Time_L4" class="Str"("Val(Sgnl)"=w1829) -> ()  [unwired: 2 in, 2 out]
            n188 = property on="Start Time_Currents_Graphs" class="Str"("Val(Sgnl)"=w1829) -> ()  [unwired: 2 in, 2 out]
            n189 = property on="Start Time_T_P" class="Str"("Val(Sgnl)"=w1829) -> ()  [unwired: 2 in, 2 out]
          }
        }
        n190 = Absolute Value(x=w241) -> (abs(x)=→"S8-2R R_G1":dbl)
        n191 = Absolute Value(x=w238) -> (abs(x)=→"S8-2L R_G1":dbl)
        n192 = Absolute Value(x=w235) -> (abs(x)=→"S7-2R R_G1":dbl)
        n193 = Absolute Value(x=w234) -> (abs(x)=→"S7-2L R_G1":dbl)
        n194 = Absolute Value(x=w239) -> (abs(x)=→"S6-2R R_G1":dbl)
        n195 = Absolute Value(x=w230) -> (abs(x)=→"S6-2L R_G1":dbl)
        n196 = local read "Presure [Pa]"() -> (w1526:i32)
        n197 = Unbundle("Limits") -> (w952:dbl, w948:dbl)
        n198 = Unbundle("Limits 2") -> (w342:dbl, w344:dbl)
        n199 = local read "E8-2R V"() -> (w276:dbl)
        n200 = local read "E7-2R V"() -> (w280:dbl)
        n201 = local read "E6-2R V"() -> (w283:dbl)
        n202 = local read "E8-2L V"() -> (w278:dbl)
        n203 = local read "E7-2L V"() -> (w287:dbl)
        n204 = local read "E6-2L V"() -> (w285:dbl)
        n205 = local read "E8-2R I"() -> (w277:dbl)
        n206 = local read "E7-2R I"() -> (w281:dbl)
        n207 = local read "E6-2R I"() -> (w284:dbl)
        n208 = local read "E8-2L I"() -> (w279:dbl)
        n209 = local read "E7-2L I"() -> (w282:dbl)
        n210 = local read "E6-2L I"() -> (w286:dbl)
        n211 = local read "S8-2R V"() -> (→"L1_S8-2R_ind":dbl)
        n212 = local read "S7-2R V"() -> (→"L1_S7-2R_ind":dbl)
        n213 = local read "S6-2R V"() -> (→"L1_S6-2R_ind":dbl)
        n214 = local read "S8-1R V"() -> (→"L2_S8-1R_ind":dbl)
        n215 = local read "S7-1R V"() -> (→"L2_S7-1R_ind":dbl)
        n216 = local read "S6-1R V"() -> (→"L2_S6-1R_ind":dbl)
        n217 = local read "S8-2L V"() -> (→"L1_S8-2L_ind":dbl)
        n218 = local read "S7-2L V"() -> (→"L1_S7-2L_ind":dbl)
        n219 = local read "S6-2L V"() -> (→"L1_S6-2L_ind":dbl)
        n220 = local read "S8-1L V"() -> (→"L2_S8-1L_ind":dbl)
        n221 = local read "S7-1L V"() -> (→"L2_S7-1L_ind":dbl)
        n222 = local read "S6-1L V"() -> (→"L2_S6-1L_ind":dbl)
        n223 = Get Date/Time In Seconds() -> (seconds since 1Jan1904=w442:timestamp)
        n224 = Seconds To Date/Time(time stamp (now)=w442) -> (date time rec=w1142:T4)  [unwired: 1 in]
        n225 = Unbundle By Name(w1142) -> ("fractional second"=w1128:dbl, "second"=w1138:i32, "minute"=w1137:i32, "hour"=w1136:i32, "day of month"=w1135:i32, "month"=w1134:i32, "year"=w1133:i32, "day of week"=w1132:i32, "day of year"=w1131:i32, "DST"=w1130:i32)
        n226 = Build Array(w1220, w1219, w1218, w1217, w1216, w1213) -> (w1212:dbl[][])
        n227 = Build Array(w1198, w1197, w1196, w1195, w1194, w1193) -> (w1192:dbl[][])
        n228 = Build Array(w1177, w1176, w1175, w1174, w1173, w1172) -> (w1171:dbl[][])
        n229 = Build Array(w1160, w1159, w1158, w1157, w1156, w1155) -> (w1154:dbl[][])
        n230 = Subtract(x=w1138, y=w1127) -> (x-y=w1139:i32)
        n231 = local read "S6-2L I"() -> (w985:dbl)
        n232 = local read "S6-2R I"() -> (w984:dbl)
        n233 = local read "S7-2L I"() -> (w983:dbl)
        n234 = local read "S7-2R I"() -> (w981:dbl)
        n235 = local read "S8-2L I"() -> (w973:dbl)
        n236 = local read "S8-2R I"() -> (w972:dbl)
        n237 = local read "S6-2L I"() -> (w317:dbl)
        n238 = local read "S6-2R I"() -> (w318:dbl)
        n239 = local read "S7-2L I"() -> (w319:dbl)
        n240 = local read "S7-2R I"() -> (w320:dbl)
        n241 = local read "S8-2L I"() -> (w321:dbl)
        n242 = local read "S8-2R I"() -> (w322:dbl)
        n243 = Build Array(w1547, w1546, w1545, w1544, w1543, w1542) -> (w1524:dbl[][])
        n244 = Build Array(w1522, w1521, w1520, w1519, w1518, w1517) -> (w1516:dbl[][])
        n245 = Build Array(w1514, w1513, w1512, w1511, w1510, w1509) -> (w1515:dbl[][])
        n246 = Build Array(w1506, w1505, w1504, w1503, w1502, w1501) -> (w1507:dbl[][])
        n247 = Build Array(w1496, w1495, w1494, w1493, w1492, w1491) -> (w1500:dbl[][])
        n248 = Build Array(w1490, w1489, w1488, w1487, w1486, w1485) -> (w1499:dbl[][])
        n249 = Build Array(w1484, w1483, w1482, w1481, w1480, w1479) -> (w1498:dbl[][])
        n250 = Build Array(w1478, w1477, w1476, w1475, w1474, w1473) -> (w1497:dbl[][])
        n251 = Subtract(x=w1137, y=w1126) -> (x-y=w1140:i32)
        n252 = Build Array (concatenate)(w1548, w442) -> (w1347:timestamp[])
        n253 = Build Array(w868, w869, w870, w871, w872, w875) -> (w876:dbl[][])
        n254 = Build Array(w890, w891, w892, w893, w894, w895) -> (w896:dbl[][])
        n255 = Build Array(w911, w912, w913, w914, w915, w916) -> (w917:dbl[][])
        n256 = Build Array(w928, w929, w930, w931, w932, w933) -> (w934:dbl[][])
        n257 = Divide(x=w952, y=w947) -> (x/y=w951:dbl)
        n258 = Divide(x=w948, y=w947) -> (x/y=w953:dbl)
        n259 = Divide(x=w342, y=w292) -> (x/y=w343:dbl)
        n260 = Divide(x=w344, y=w292) -> (x/y=w341:dbl)
        n261 = Divide(x=w276, y=w277) -> (x/y=w226:dbl)
        n262 = Divide(x=w278, y=w279) -> (x/y=w225:dbl)
        n263 = Divide(x=w280, y=w281) -> (x/y=w224:dbl)
        n264 = Divide(x=w287, y=w282) -> (x/y=w223:dbl)
        n265 = Divide(x=w283, y=w284) -> (x/y=w222:dbl)
        n266 = Divide(x=w285, y=w286) -> (x/y=w228:dbl)
        n267 = Subtract(x=w1136, y=w1125) -> (x-y=w1141:i32)
        n268 = Build Array(w682, w683, w684, w685, w686, w687) -> (w699:dbl[][])
        n269 = Build Array(w700, w701, w702, w703, w704, w705) -> (w706:dbl[][])
        n270 = Build Array(w708, w709, w710, w711, w712, w713) -> (w707:dbl[][])
        n271 = Build Array(w715, w716, w717, w718, w719, w720) -> (w714:dbl[][])
        n272 = Build Array(w725, w726, w727, w728, w729, w730) -> (w721:dbl[][])
        n273 = Build Array(w731, w732, w733, w734, w735, w736) -> (w722:dbl[][])
        n274 = Build Array(w737, w738, w739, w740, w741, w742) -> (w723:dbl[][])
        n275 = Build Array(w743, w744, w745, w746, w747, w748) -> (w724:dbl[][])
        n276 = Compound Arithmetic op=OR("Full_Clear_1", "Full_Clear_2", "Full_Clear_3", "Full_Clear_4", "Full_Clear_5") -> (w1102:bool)
        n277 = Absolute Value(x=w226) -> (abs(x)=→"E8-1R R_G1":dbl)
        n278 = Absolute Value(x=w225) -> (abs(x)=→"E8-1L R_G1":dbl)
        n279 = Absolute Value(x=w224) -> (abs(x)=→"E7-1R R_G1":dbl)
        n280 = Absolute Value(x=w223) -> (abs(x)=→"E7-1L R_G1":dbl)
        n281 = Absolute Value(x=w222) -> (abs(x)=→"E6-1R R_G1":dbl)
        n282 = Absolute Value(x=w228) -> (abs(x)=→"E6-1L R_G1":dbl)
        n283 = local read "Temperature [C]"() -> (w698:dbl)
        n284 = Bundle("fractional second"=w1128, w1139, w1140, w1141, "day of month"=w1135, "month"=w1134, "year"=w1133, "day of week"=w1132, "day of year"=w1131, "DST"=w1130) -> (w1129:T6)  [unwired: 1 in]
        n285 = local read "Presure [Pa]"() -> (w697:i32)
        n286 = call "Level.vi"("Y_Lev_max"=w951, "IN"=w985, "G_Lev_max"=w953) -> ("R"=→"6-L_R_L1":bool, "Y"=→"6-L_Y_L1":bool, "G"=→"6-L_G_L1":bool)
        n287 = call "Level.vi"("Y_Lev_max"=w951, "IN"=w984, "G_Lev_max"=w953) -> ("R"=→"6-R_R_L1":bool, "Y"=→"6-R_Y_L1":bool, "G"=→"6-R_G_L1":bool)
        n288 = call "Level.vi"("Y_Lev_max"=w951, "IN"=w983, "G_Lev_max"=w953) -> ("R"=→"7-L_R_L1":bool, "Y"=→"7-L_Y_L1":bool, "G"=→"7-L_G_L1":bool)
        n289 = call "Level.vi"("Y_Lev_max"=w951, "IN"=w981, "G_Lev_max"=w953) -> ("R"=→"7-R_R_L1":bool, "Y"=→"7-R_Y_L1":bool, "G"=→"7-R_G_L1":bool)
        n290 = call "Level.vi"("Y_Lev_max"=w951, "IN"=w973, "G_Lev_max"=w953) -> ("R"=→"8-L_R_L1":bool, "Y"=→"8-L_Y_L1":bool, "G"=→"8-L_G_L1":bool)
        n291 = call "Level.vi"("Y_Lev_max"=w951, "IN"=w972, "G_Lev_max"=w953) -> ("R"=→"8-R_R_L1":bool, "Y"=→"8-R_Y_L1":bool, "G"=→"8-R_G_L1":bool)
        n292 = call "Level.vi"("Y_Lev_max"=w343, "IN"=w317, "G_Lev_max"=w341) -> ("R"=→"6-L_R_L1 2":bool, "Y"=→"6-L_Y_L1 2":bool, "G"=→"6-L_G_L1 2":bool)
        n293 = call "Level.vi"("Y_Lev_max"=w343, "IN"=w318, "G_Lev_max"=w341) -> ("R"=→"6-R_R_L1 2":bool, "Y"=→"6-R_Y_L1 2":bool, "G"=→"6-R_G_L1 2":bool)
        n294 = call "Level.vi"("Y_Lev_max"=w343, "IN"=w319, "G_Lev_max"=w341) -> ("R"=→"7-L_R_L1 2":bool, "Y"=→"7-L_Y_L1 2":bool, "G"=→"7-L_G_L1 2":bool)
        n295 = call "Level.vi"("Y_Lev_max"=w343, "IN"=w320, "G_Lev_max"=w341) -> ("R"=→"7-R_R_L1 2":bool, "Y"=→"7-R_Y_L1 2":bool, "G"=→"7-R_G_L1 2":bool)
        n296 = call "Level.vi"("Y_Lev_max"=w343, "IN"=w321, "G_Lev_max"=w341) -> ("R"=→"8-L_R_L1 2":bool, "Y"=→"8-L_Y_L1 2":bool, "G"=→"8-L_G_L1 2":bool)
        n297 = call "Level.vi"("Y_Lev_max"=w343, "IN"=w322, "G_Lev_max"=w341) -> ("R"=→"8-R_R_L1 2":bool, "Y"=→"8-R_Y_L1 2":bool, "G"=→"8-R_G_L1 2":bool)
        n298 = Date/Time To Seconds(2:w1129) -> (0:w590:timestamp)  [unwired: 1 in]
        n299 = Build Array (concatenate)(w1143, w590) -> (w589:timestamp[])
        n300 = local read "S8-1R V"() -> (w215:dbl)
        n301 = local read "S7-1R V"() -> (w245:dbl)
        n302 = local read "S6-1R V"() -> (w249:dbl)
        n303 = local read "S8-1L V"() -> (w243:dbl)
        n304 = local read "S7-1L V"() -> (w247:dbl)
        n305 = local read "S6-1L V"() -> (w251:dbl)
        n306 = local read "S8-1R I"() -> (w242:dbl)
        n307 = local read "S7-1R I"() -> (w246:dbl)
        n308 = local read "S6-1R I"() -> (w250:dbl)
        n309 = local read "S8-1L I"() -> (w244:dbl)
        n310 = local read "S7-1L I"() -> (w248:dbl)
        n311 = local read "S6-1L I"() -> (w252:dbl)
        n312 = local read "E8-2R V"() -> (→"L3_E8-2R_ind":dbl)
        n313 = local read "E7-2R V"() -> (→"L3_E7-2R_ind":dbl)
        n314 = local read "E6-2R V"() -> (→"L3_E6-2R_ind":dbl)
        n315 = local read "E8-1R V"() -> (→"L4_E8-1R_ind":dbl)
        n316 = local read "E7-1R V"() -> (→"L4_E7-1R_ind":dbl)
        n317 = local read "E6-1R V"() -> (→"L4_E6-1R_ind":dbl)
        n318 = local read "E8-2L V"() -> (→"L3_E8-2L_ind":dbl)
        n319 = local read "E7-2L V"() -> (→"L3_E7-2L_ind":dbl)
        n320 = local read "E6-2L V"() -> (→"L3_E6-2L_ind":dbl)
        n321 = local read "E8-1L V"() -> (→"L4_E8-1L_ind":dbl)
        n322 = local read "E7-1L V"() -> (→"L4_E7-1L_ind":dbl)
        n323 = local read "E6-1L V"() -> (→"L4_E6-1L_ind":dbl)
        n324 = Divide(x=w215, y=w242) -> (x/y=w214:dbl)
        n325 = Divide(x=w243, y=w244) -> (x/y=w217:dbl)
        n326 = Divide(x=w245, y=w246) -> (x/y=w212:dbl)
        n327 = Divide(x=w247, y=w248) -> (x/y=w209:dbl)
        n328 = Divide(x=w249, y=w250) -> (x/y=w208:dbl)
        n329 = Divide(x=w251, y=w252) -> (x/y=w205:dbl)
        n330 = Absolute Value(x=w214) -> (abs(x)=→"S8-1R R_G1":dbl)
        n331 = Absolute Value(x=w217) -> (abs(x)=→"S8-1L R_G1":dbl)
        n332 = Absolute Value(x=w212) -> (abs(x)=→"S7-1R R_G1":dbl)
        n333 = Absolute Value(x=w209) -> (abs(x)=→"S7-1L R_G1":dbl)
        n334 = Absolute Value(x=w208) -> (abs(x)=→"S6-1R R_G1":dbl)
        n335 = Absolute Value(x=w205) -> (abs(x)=→"S6-1L R_G1":dbl)
        n336 = local read "S6-1L I"() -> (w966:dbl)
        n337 = local read "S6-1R I"() -> (w971:dbl)
        n338 = local read "S7-1L I"() -> (w970:dbl)
        n339 = local read "S7-1R I"() -> (w969:dbl)
        n340 = local read "S8-1L I"() -> (w968:dbl)
        n341 = local read "S8-1R I"() -> (w967:dbl)
        n342 = local read "S6-1L I"() -> (w328:dbl)
        n343 = local read "S6-1R I"() -> (w323:dbl)
        n344 = local read "S7-1L I"() -> (w324:dbl)
        n345 = local read "S7-1R I"() -> (w325:dbl)
        n346 = local read "S8-1L I"() -> (w326:dbl)
        n347 = local read "S8-1R I"() -> (w327:dbl)
        n348 = Compound Arithmetic op=OR("Full_Clear_1 2", "Full_Clear_2 2", "Full_Clear_3 2", "Full_Clear_4 2", "Full_Clear_5 2") -> (w681:bool)
        n349 = Build Array (concatenate)(w1287, w1283) -> (w1351:i32[])
        n350 = Build Array (concatenate)(w1286, w1107) -> (w1349:dbl[])
        n351 = local read "E8-2R V"() -> (w264:dbl)
        n352 = local read "E7-2R V"() -> (w268:dbl)
        n353 = local read "E6-2R V"() -> (w272:dbl)
        n354 = local read "E8-2L V"() -> (w266:dbl)
        n355 = local read "E7-2L V"() -> (w270:dbl)
        n356 = local read "E6-2L V"() -> (w274:dbl)
        n357 = local read "E8-2R I"() -> (w265:dbl)
        n358 = local read "E7-2R I"() -> (w269:dbl)
        n359 = local read "E6-2R I"() -> (w273:dbl)
        n360 = local read "E8-2L I"() -> (w267:dbl)
        n361 = local read "E7-2L I"() -> (w271:dbl)
        n362 = local read "E6-2L I"() -> (w275:dbl)
        n363 = call "Level.vi"("Y_Lev_max"=w951, "IN"=w966, "G_Lev_max"=w953) -> ("R"=→"6-L_R_L2":bool, "Y"=→"6-L_Y_L2":bool, "G"=→"6-L_G_L2":bool)
        n364 = call "Level.vi"("Y_Lev_max"=w951, "IN"=w971, "G_Lev_max"=w953) -> ("R"=→"6-R_R_L2":bool, "Y"=→"6-R_Y_L2":bool, "G"=→"6-R_G_L2":bool)
        n365 = call "Level.vi"("Y_Lev_max"=w951, "IN"=w970, "G_Lev_max"=w953) -> ("R"=→"7-L_R_L2":bool, "Y"=→"7-L_Y_L2":bool, "G"=→"7-L_G_L2":bool)
        n366 = call "Level.vi"("Y_Lev_max"=w951, "IN"=w969, "G_Lev_max"=w953) -> ("R"=→"7-R_R_L2":bool, "Y"=→"7-R_Y_L2":bool, "G"=→"7-R_G_L2":bool)
        n367 = call "Level.vi"("Y_Lev_max"=w951, "IN"=w968, "G_Lev_max"=w953) -> ("R"=→"8-L_R_L2":bool, "Y"=→"8-L_Y_L2":bool, "G"=→"8-L_G_L2":bool)
        n368 = call "Level.vi"("Y_Lev_max"=w951, "IN"=w967, "G_Lev_max"=w953) -> ("R"=→"8-R_R_L2":bool, "Y"=→"8-R_Y_L2":bool, "G"=→"8-R_G_L2":bool)
        n369 = call "Level.vi"("Y_Lev_max"=w343, "IN"=w328, "G_Lev_max"=w341) -> ("R"=→"6-L_R_L2 2":bool, "Y"=→"6-L_Y_L2 2":bool, "G"=→"6-L_G_L2 2":bool)
        n370 = call "Level.vi"("Y_Lev_max"=w343, "IN"=w323, "G_Lev_max"=w341) -> ("R"=→"6-R_R_L2 2":bool, "Y"=→"6-R_Y_L2 2":bool, "G"=→"6-R_G_L2 2":bool)
        n371 = call "Level.vi"("Y_Lev_max"=w343, "IN"=w324, "G_Lev_max"=w341) -> ("R"=→"7-L_R_L2 2":bool, "Y"=→"7-L_Y_L2 2":bool, "G"=→"7-L_G_L2 2":bool)
        n372 = call "Level.vi"("Y_Lev_max"=w343, "IN"=w325, "G_Lev_max"=w341) -> ("R"=→"7-R_R_L2 2":bool, "Y"=→"7-R_Y_L2 2":bool, "G"=→"7-R_G_L2 2":bool)
        n373 = call "Level.vi"("Y_Lev_max"=w343, "IN"=w326, "G_Lev_max"=w341) -> ("R"=→"8-L_R_L2 2":bool, "Y"=→"8-L_Y_L2 2":bool, "G"=→"8-L_G_L2 2":bool)
        n374 = call "Level.vi"("Y_Lev_max"=w343, "IN"=w327, "G_Lev_max"=w341) -> ("R"=→"8-R_R_L2 2":bool, "Y"=→"8-R_Y_L2 2":bool, "G"=→"8-R_G_L2 2":bool)
        n375 = Bundle(w589, w1349) -> (→"Temperature Graph":cluster{timestamp[], dbl[]})  [unwired: 1 in]
        n376 = Bundle(w589, w1351) -> (→"Presure Graph":cluster{timestamp[], i32[]})  [unwired: 1 in]
        n377 = Divide(x=w264, y=w265) -> (x/y=w199:dbl)
        n378 = Divide(x=w266, y=w267) -> (x/y=w200:dbl)
        n379 = Divide(x=w268, y=w269) -> (x/y=w201:dbl)
        n380 = Divide(x=w270, y=w271) -> (x/y=w202:dbl)
        n381 = Divide(x=w272, y=w273) -> (x/y=w203:dbl)
        n382 = Divide(x=w274, y=w275) -> (x/y=w204:dbl)
        n383 = Absolute Value(x=w199) -> (abs(x)=→"E8-2R R_G1":dbl)
        n384 = Absolute Value(x=w200) -> (abs(x)=→"E8-2L R_G1":dbl)
        n385 = Absolute Value(x=w201) -> (abs(x)=→"E7-2R R_G1":dbl)
        n386 = Absolute Value(x=w202) -> (abs(x)=→"E7-2L R_G1":dbl)
        n387 = Absolute Value(x=w203) -> (abs(x)=→"E6-2R R_G1":dbl)
        n388 = Absolute Value(x=w204) -> (abs(x)=→"E6-2L R_G1":dbl)
        n389 = property on="IP Address" class="Str"() -> ("Value"=w168:string)  [unwired: 2 in, 2 out]
        n390 = property on="Username" class="Str"() -> ("Value"=w169:string)  [unwired: 2 in, 2 out]
        n391 = property on="Password" class="Str"() -> ("Value"=w170:string)  [unwired: 2 in, 2 out]
        n392 = property on="Group 1" class="Ring (strict)"() -> ("Value"=w171:u16)  [unwired: 2 in, 2 out]
        n393 = property on="Group 2" class="Ring (strict)"() -> ("Value"=w172:u16)  [unwired: 2 in, 2 out]
        n394 = property on="Group 1 log name" class="Str"() -> ("Value"=w173:string)  [unwired: 2 in, 2 out]
        n395 = property on="Group 2 log name" class="Str"() -> ("Value"=w174:string)  [unwired: 2 in, 2 out]
        n396 = property on="COM Port" class="VISAName"() -> ("Value"=w175:refnum<visa-resource-name>)  [unwired: 2 in, 2 out]
        n397 = property on="Delay [s]" class="DigNum (strict)"() -> ("Value"=w176:dbl)  [unwired: 2 in, 2 out]
        n398 = property on="Tempt-Presure-on-off" class="Bool (strict)"() -> ("Value"=w177:bool)  [unwired: 2 in, 2 out]
        n399 = property on="Graphs bachground Color" class="ColBox"() -> ("Value"=w178:u32)  [unwired: 2 in, 2 out]
        n400 = property on="Pages Colors" class="Arr (strict)"() -> ("Value"=w179:u32[])  [unwired: 2 in, 2 out]
        n401 = local read "E6-2L I"() -> (w965:dbl)
        n402 = local read "E6-2R I"() -> (w962:dbl)
        n403 = local read "E7-2L I"() -> (w961:dbl)
        n404 = local read "E7-2R I"() -> (w960:dbl)
        n405 = local read "E8-2L I"() -> (w964:dbl)
        n406 = local read "E8-2R I"() -> (w963:dbl)
        n407 = local read "E6-2L I"() -> (w329:dbl)
        n408 = local read "E6-2R I"() -> (w332:dbl)
        n409 = local read "E7-2L I"() -> (w333:dbl)
        n410 = local read "E7-2R I"() -> (w334:dbl)
        n411 = local read "E8-2L I"() -> (w330:dbl)
        n412 = local read "E8-2R I"() -> (w331:dbl)
        n413 = call "Level.vi"("Y_Lev_max"=w951, "IN"=w965, "G_Lev_max"=w953) -> ("R"=→"6-L_R_L3":bool, "Y"=→"6-L_Y_L3":bool, "G"=→"6-L_G_L3":bool)
        n414 = call "Level.vi"("Y_Lev_max"=w951, "IN"=w962, "G_Lev_max"=w953) -> ("R"=→"6-R_R_L3":bool, "Y"=→"6-R_Y_L3":bool, "G"=→"6-R_G_L3":bool)
        n415 = call "Level.vi"("Y_Lev_max"=w951, "IN"=w961, "G_Lev_max"=w953) -> ("R"=→"7-L_R_L3":bool, "Y"=→"7-L_Y_L3":bool, "G"=→"7-L_G_L3":bool)
        n416 = call "Level.vi"("Y_Lev_max"=w951, "IN"=w960, "G_Lev_max"=w953) -> ("R"=→"7-R_R_L3":bool, "Y"=→"7-R_Y_L3":bool, "G"=→"7-R_G_L3":bool)
        n417 = call "Level.vi"("Y_Lev_max"=w951, "IN"=w964, "G_Lev_max"=w953) -> ("R"=→"8-L_R_L3":bool, "Y"=→"8-L_Y_L3":bool, "G"=→"8-L_G_L3":bool)
        n418 = call "Level.vi"("Y_Lev_max"=w951, "IN"=w963, "G_Lev_max"=w953) -> ("R"=→"8-R_R_L3":bool, "Y"=→"8-R_Y_L3":bool, "G"=→"8-R_G_L3":bool)
        n419 = call "Level.vi"("Y_Lev_max"=w343, "IN"=w329, "G_Lev_max"=w341) -> ("R"=→"6-L_R_L3 2":bool, "Y"=→"6-L_Y_L3 2":bool, "G"=→"6-L_G_L3 2":bool)
        n420 = call "Level.vi"("Y_Lev_max"=w343, "IN"=w332, "G_Lev_max"=w341) -> ("R"=→"6-R_R_L3 2":bool, "Y"=→"6-R_Y_L3 2":bool, "G"=→"6-R_G_L3 2":bool)
        n421 = call "Level.vi"("Y_Lev_max"=w343, "IN"=w333, "G_Lev_max"=w341) -> ("R"=→"7-L_R_L3 2":bool, "Y"=→"7-L_Y_L3 2":bool, "G"=→"7-L_G_L3 2":bool)
        n422 = call "Level.vi"("Y_Lev_max"=w343, "IN"=w334, "G_Lev_max"=w341) -> ("R"=→"7-R_R_L3 2":bool, "Y"=→"7-R_Y_L3 2":bool, "G"=→"7-R_G_L3 2":bool)
        n423 = call "Level.vi"("Y_Lev_max"=w343, "IN"=w330, "G_Lev_max"=w341) -> ("R"=→"8-L_R_L3 2":bool, "Y"=→"8-L_Y_L3 2":bool, "G"=→"8-L_G_L3 2":bool)
        n424 = call "Level.vi"("Y_Lev_max"=w343, "IN"=w331, "G_Lev_max"=w341) -> ("R"=→"8-R_R_L3 2":bool, "Y"=→"8-R_Y_L3 2":bool, "G"=→"8-R_G_L3 2":bool)
        n425 = property on="logs_directory_path" class="Path"() -> ("Value"=w162:path)  [unwired: 2 in, 2 out]
        n426 = Boolean To (0,1)(Boolean="Logarithm scale 2") -> (0, 1=w591:i16)
        n427 = case shown="0, Default" "Group 1" {
          tunnel: [0 0 0 1 1 1 2 2 2 3 3 3] -> w166
          tunnel: [1 2 3 0 2 3 0 1 3 0 1 2] -> w165
          frame 0, Default {
          }
          frame 1 {
          }
          frame 2 {
          }
          frame 3 {
          }
          frame 4 {
          }
          frame 5 {
          }
          frame 6 {
          }
          frame 7 {
          }
          frame 8 {
          }
          frame 9 {
          }
          frame 10 {
          }
          frame 11 {
          }
        }
        n428 = case shown="0, Default" "Group 2" {
          tunnel: [0 0 0 1 1 1 2 2 2 3 3 3] -> w164
          tunnel: [1 2 3 0 2 3 0 1 3 0 1 2] -> w163
          frame 0, Default {
          }
          frame 1 {
          }
          frame 2 {
          }
          frame 3 {
          }
          frame 4 {
          }
          frame 5 {
          }
          frame 6 {
          }
          frame 7 {
          }
          frame 8 {
          }
          frame 9 {
          }
          frame 10 {
          }
          frame 11 {
          }
        }
        n429 = property on="L1 (St-2) -V 2" class="XYGraph (strict)"("BG Color"="Graphs bachground Color") -> ()  [unwired: 2 in, 2 out]
        n430 = property on="L1 (St-2) -I 2" class="XYGraph (strict)"("BG Color"="Graphs bachground Color") -> ()  [unwired: 2 in, 2 out]
        n431 = property on="L1 (St-2) -V" class="XYGraph (strict)"("BG Color"="Graphs bachground Color") -> ()  [unwired: 2 in, 2 out]
        n432 = property on="L1 (St-2) -I" class="XYGraph (strict)"("BG Color"="Graphs bachground Color") -> ()  [unwired: 2 in, 2 out]
        n433 = property on="L1 (St-2)" class="XYGraph (strict)"("YScale.Mapping Mode"=w591) -> ()  [unwired: 2 in, 2 out]
        n434 = property on="L2 (St-1)" class="XYGraph (strict)"("YScale.Mapping Mode"=w591) -> ()  [unwired: 2 in, 2 out]
        n435 = property on="L3 (Eta-2 )" class="XYGraph (strict)"("YScale.Mapping Mode"=w591) -> ()  [unwired: 2 in, 2 out]
        n436 = property on="L4 (Eta-1)" class="XYGraph (strict)"("YScale.Mapping Mode"=w591) -> ()  [unwired: 2 in, 2 out]
        n437 = Boolean To (0,1)(Boolean="Logarithm scale 6") -> (0, 1=w659:i16)
        n438 = Build Array(w166, w165, w164, w163) -> (w181:i32[])
        n439 = call "Read_Current_values_with_slots_select.vi"("error in"=w1529, "Board_index"=w181, "handle"=w1448) -> ("error out"=w1449:errorcluster, "Status"=w443:bool[][], "IMon--VMon"=w667:T7)  [unwired: 3 out]
        n440 = call-poly <vilib>:"Matrix To Array.vi"("Real Matrix"=w667) -> ("Real 2D Array"=w1539:dbl[][])
        n441 = call-poly <vilib>:"Matrix To Array.vi"("Real Matrix"=w667) -> ("Real 2D Array"=w690:dbl[][])
        n442 = Transpose 2D Array(2D array=w1539) -> (transposed array=w1541:dbl[][])
        n443 = Transpose 2D Array(2D array=w443) -> (transposed array=w1530:bool[][])
        n444 = Transpose 2D Array(2D array=w443) -> (transposed array=w450:bool[][])
        n445 = Transpose 2D Array(2D array=w690) -> (transposed array=w688:dbl[][])
        n446 = Index Array(array=w1541, index (row) #1=0 ("index (row)"), index (row) #2=1 ("index (row)"), index (row) #3=2 ("index (row)"), index (row) #4=3 ("index (row)")) -> (element #1=w1534:dbl[], element #2=w1113:dbl[], element #3=w1535:dbl[], element #4=w1112:dbl[])  [unwired: 4 in]
        n447 = Index Array(array=w1530, index (row) #1=0 ("index (row)"), index (row) #2=1 ("index (row)")) -> (element #1=w1453:bool[], element #2=w1450:bool[])  [unwired: 2 in]
        n448 = Index Array(array=w450, index (row) #1=2 ("index (row)"), index (row) #2=3 ("index (row)")) -> (element #1=w447:bool[], element #2=w444:bool[])  [unwired: 2 in]
        n449 = Index Array(array=w688, index (row) #1=4 ("index (row)"), index (row) #2=5 ("index (row)"), index (row) #3=6 ("index (row)"), index (row) #4=7 ("index (row)")) -> (element #1=w695:dbl[], element #2=w938:dbl[], element #3=w694:dbl[], element #4=w939:dbl[])  [unwired: 4 in]
        n450 = Build Array (concatenate)(w1534, w1535) -> (w189:dbl[])
        n451 = Build Array (concatenate)(w1113, w1112) -> (w596:dbl[])
        n452 = Array Subset(array=w1453, index=0, length=w1454) -> (w561:bool[])
        n453 = Index Array(array=w561) -> (element #1=w1090:bool, element #2=w1089:bool, element #3=w1085:bool, element #4=w1088:bool, element #5=w1087:bool, element #6=w1086:bool)  [unwired: 6 in]
        n454 = Not(x=w1090) -> (.not. x?=→"8-R_Gr_L1":bool)
        n455 = Not(x=w1089) -> (.not. x?=→"8-L_Gr_L1":bool)
        n456 = Not(x=w1085) -> (.not. x?=→"7-R_Gr_L1":bool)
        n457 = Not(x=w1088) -> (.not. x?=→"7-L_Gr_L1":bool)
        n458 = Not(x=w1087) -> (.not. x?=→"6-R_Gr_L1":bool)
        n459 = Not(x=w1086) -> (.not. x?=→"6-L_Gr_L1":bool)
        n460 = Array Subset(array=w1453, index=w1454) -> (w588:bool[])  [unwired: 1 in]
        n461 = Array Subset(array=w1450, index=0, length=w1452) -> (w587:bool[])
        n462 = Array Subset(array=w1450, index=w1452) -> (w586:bool[])  [unwired: 1 in]
        n463 = Array Subset(array=w447, index=0, length=w448) -> (w291:bool[])
        n464 = Index Array(array=w291) -> (element #1=w293:bool, element #2=w294:bool, element #3=w298:bool, element #4=w295:bool, element #5=w296:bool, element #6=w297:bool)  [unwired: 6 in]
        n465 = Not(x=w293) -> (.not. x?=→"8-R_Gr_L1 2":bool)
        n466 = Not(x=w294) -> (.not. x?=→"8-L_Gr_L1 2":bool)
        n467 = Not(x=w298) -> (.not. x?=→"7-R_Gr_L1 2":bool)
        n468 = Not(x=w295) -> (.not. x?=→"7-L_Gr_L1 2":bool)
        n469 = Not(x=w296) -> (.not. x?=→"6-R_Gr_L1 2":bool)
        n470 = Not(x=w297) -> (.not. x?=→"6-L_Gr_L1 2":bool)
        n471 = Array Subset(array=w447, index=w448) -> (w290:bool[])  [unwired: 1 in]
        n472 = Array Subset(array=w444, index=0, length=w446) -> (w289:bool[])
        n473 = Array Subset(array=w444, index=w446) -> (w288:bool[])  [unwired: 1 in]
        n474 = Build Array (concatenate)(w695, w694) -> (w186:dbl[])
        n475 = Build Array (concatenate)(w938, w939) -> (w680:dbl[])
        n476 = call "offsets_R-W.vi"("Offset_R/W"="Offsets", "parameter"="Offset_Group1", "Real IMon"=w189) -> ("corection IMon"=w188:dbl[])
        n477 = call "offsets_R-W.vi"("Offset_R/W"="Offsets 2", "parameter"="Offset_Group2", "Real IMon"=w186) -> ("corection IMon"=w184:dbl[])
        n478 = Array Subset(array=w188, index=0, length=w1468) -> (w1106:dbl[])
        n479 = Array Subset(array=w188, index=w1468, length=w1468) -> (w1105:dbl[])
        n480 = Array Subset(array=w596, index=0, length=w1110) -> (w1109:dbl[])
        n481 = Array Subset(array=w596, index=w1110) -> (w1108:dbl[])  [unwired: 1 in]
        n482 = Array Subset(array=w184, index=0, length=w749) -> (w944:dbl[])
        n483 = Array Subset(array=w184, index=w749, length=w749) -> (w945:dbl[])
        n484 = Array Subset(array=w680, index=0, length=w941) -> (w942:dbl[])
        n485 = Array Subset(array=w680, index=w941) -> (w943:dbl[])  [unwired: 1 in]
        n486 = Array Subset(array=w1106, index=w1467, length=w1466) -> (w1211:dbl[])
        n487 = call "Channel_plots.vi"("Current time"=w589, "In Channels"=w1212, "Input Channels"=w1211) -> ("output graph"=→"L1 (St-2)":T2, "out Ch 1"=w1230:dbl[], "out Ch 6"=w1215:dbl[], "out Ch 2"=w1228:dbl[], "out Ch 3"=w1226:dbl[], "out Ch 4"=w1224:dbl[], "out Ch 5"=w1222:dbl[])
        n488 = call "Channel_plots.vi"("Current time"=w589, "In Channels"=w1516, "Input Channels"=w1211) -> ("output graph"=→"L1 (St-2) -I":T2, "out Ch 1"=w1435:dbl[], "out Ch 6"=w1425:dbl[], "out Ch 2"=w1433:dbl[], "out Ch 3"=w1431:dbl[], "out Ch 4"=w1429:dbl[], "out Ch 5"=w1427:dbl[])
        n489 = Array Subset(array=w1106, index=w1466) -> (w1151:dbl[])  [unwired: 1 in]
        n490 = call "Channel_plots.vi"("Current time"=w589, "In Channels"=w1192, "Input Channels"=w1151) -> ("output graph"=→"L2 (St-1)":T2, "out Ch 1"=w1210:dbl[], "out Ch 6"=w1200:dbl[], "out Ch 2"=w1208:dbl[], "out Ch 3"=w1206:dbl[], "out Ch 4"=w1204:dbl[], "out Ch 5"=w1202:dbl[])
        n491 = call "Channel_plots.vi"("Current time"=w589, "In Channels"=w1507, "Input Channels"=w1151) -> ("output graph"=→"L2 (St-1) -I":T2, "out Ch 1"=w1411:dbl[], "out Ch 6"=w1401:dbl[], "out Ch 2"=w1409:dbl[], "out Ch 3"=w1407:dbl[], "out Ch 4"=w1405:dbl[], "out Ch 5"=w1403:dbl[])
        n492 = Array Subset(array=w1105, index=w1467, length=w1466) -> (w1152:dbl[])
        n493 = call "Channel_plots.vi"("Current time"=w589, "In Channels"=w1171, "Input Channels"=w1152) -> ("output graph"=→"L3 (Eta-2 )":T2, "out Ch 1"=w1191:dbl[], "out Ch 6"=w1181:dbl[], "out Ch 2"=w1188:dbl[], "out Ch 3"=w1187:dbl[], "out Ch 4"=w1185:dbl[], "out Ch 5"=w1183:dbl[])
        n494 = call "Channel_plots.vi"("Current time"=w589, "In Channels"=w1499, "Input Channels"=w1152) -> ("output graph"=→"L3 (Eta-2) -I":T2, "out Ch 1"=w1387:dbl[], "out Ch 6"=w1377:dbl[], "out Ch 2"=w1385:dbl[], "out Ch 3"=w1383:dbl[], "out Ch 4"=w1381:dbl[], "out Ch 5"=w1379:dbl[])
        n495 = Array Subset(array=w1105, index=w1466) -> (w1153:dbl[])  [unwired: 1 in]
        n496 = call "Channel_plots.vi"("Current time"=w589, "In Channels"=w1154, "Input Channels"=w1153) -> ("output graph"=→"L4 (Eta-1)":T2, "out Ch 1"=w1179:dbl[], "out Ch 6"=w1162:dbl[], "out Ch 2"=w1170:dbl[], "out Ch 3"=w1168:dbl[], "out Ch 4"=w1166:dbl[], "out Ch 5"=w1164:dbl[])
        n497 = call "Channel_plots.vi"("Current time"=w589, "In Channels"=w1497, "Input Channels"=w1153) -> ("output graph"=→"L4 (Eta-1) -I":T2, "out Ch 1"=w1363:dbl[], "out Ch 6"=w1353:dbl[], "out Ch 2"=w1361:dbl[], "out Ch 3"=w1359:dbl[], "out Ch 4"=w1357:dbl[], "out Ch 5"=w1355:dbl[])
        n498 = Array Subset(array=w1109, index=w1464, length=w1465) -> (w1459:dbl[])
        n499 = call "Channel_plots.vi"("Current time"=w589, "In Channels"=w1524, "Input Channels"=w1459) -> ("output graph"=→"L1 (St-2) -V":T2, "out Ch 1"=w1447:dbl[], "out Ch 6"=w1437:dbl[], "out Ch 2"=w1445:dbl[], "out Ch 3"=w1443:dbl[], "out Ch 4"=w1441:dbl[], "out Ch 5"=w1439:dbl[])
        n500 = Array Subset(array=w1109, index=w1465) -> (w1458:dbl[])  [unwired: 1 in]
        n501 = call "Channel_plots.vi"("Current time"=w589, "In Channels"=w1515, "Input Channels"=w1458) -> ("output graph"=→"L2 (St-1) -V":T2, "out Ch 1"=w1423:dbl[], "out Ch 6"=w1413:dbl[], "out Ch 2"=w1421:dbl[], "out Ch 3"=w1419:dbl[], "out Ch 4"=w1417:dbl[], "out Ch 5"=w1415:dbl[])
        n502 = Array Subset(array=w1108, index=w1464, length=w1465) -> (w1457:dbl[])
        n503 = call "Channel_plots.vi"("Current time"=w589, "In Channels"=w1500, "Input Channels"=w1457) -> ("output graph"=→"L3 (Eta-2) -V":T2, "out Ch 1"=w1399:dbl[], "out Ch 6"=w1389:dbl[], "out Ch 2"=w1397:dbl[], "out Ch 3"=w1395:dbl[], "out Ch 4"=w1393:dbl[], "out Ch 5"=w1391:dbl[])
        n504 = Array Subset(array=w1108, index=w1465) -> (w1456:dbl[])  [unwired: 1 in]
        n505 = call "Channel_plots.vi"("Current time"=w589, "In Channels"=w1498, "Input Channels"=w1456) -> ("output graph"=→"L4 (Eta-1) -V":T2, "out Ch 1"=w1375:dbl[], "out Ch 6"=w1365:dbl[], "out Ch 2"=w1373:dbl[], "out Ch 3"=w1371:dbl[], "out Ch 4"=w1369:dbl[], "out Ch 5"=w1367:dbl[])
        n506 = case shown="True" w1102 {
          tunnel: w1447 -> [w1990 _]
          tunnel: [w1991 w2071] -> w1446
          tunnel: [w1989 w2071] -> w1444
          tunnel: w1445 -> [w1988 _]
          tunnel: [w1987 w2071] -> w1442
          tunnel: w1443 -> [w1986 _]
          tunnel: [w1985 w2071] -> w1440
          tunnel: w1441 -> [w1984 _]
          tunnel: [w1983 w2071] -> w1438
          tunnel: w1439 -> [w1982 _]
          tunnel: [w1981 w2071] -> w1436
          tunnel: w1437 -> [w1980 _]
          tunnel: w1435 -> [w1978 _]
          tunnel: [w1979 w2071] -> w1434
          tunnel: w1433 -> [w1976 _]
          tunnel: [w1977 w2071] -> w1432
          tunnel: w1431 -> [w1974 _]
          tunnel: [w1975 w2071] -> w1430
          tunnel: w1429 -> [w1972 _]
          tunnel: [w1973 w2071] -> w1428
          tunnel: w1427 -> [w1971 _]
          tunnel: [w1970 w2071] -> w1426
          tunnel: w1425 -> [w1969 _]
          tunnel: [w1968 w2071] -> w1424
          tunnel: w1423 -> [w1966 _]
          tunnel: [w1965 w2071] -> w1422
          tunnel: w1421 -> [w1963 _]
          tunnel: [w1964 w2071] -> w1420
          tunnel: w1419 -> [w1962 _]
          tunnel: [w1961 w2071] -> w1418
          tunnel: w1417 -> [w1960 _]
          tunnel: [w1959 w2071] -> w1416
          tunnel: [w1958 w2071] -> w1414
          tunnel: w1415 -> [w1957 _]
          tunnel: [w1955 w2071] -> w1412
          tunnel: w1413 -> [w1956 _]
          tunnel: [w1954 w2071] -> w1410
          tunnel: w1411 -> [w1953 _]
          tunnel: [w1952 w2071] -> w1408
          tunnel: w1409 -> [w1951 _]
          tunnel: w1407 -> [w1949 _]
          tunnel: [w1950 w2071] -> w1406
          tunnel: [w1948 w2071] -> w1404
          tunnel: w1405 -> [w1947 _]
          tunnel: w1403 -> [w1946 _]
          tunnel: [w1945 w2071] -> w1402
          tunnel: w1401 -> [w1943 _]
          tunnel: [w1944 w2071] -> w1400
          tunnel: w1399 -> [w1940 _]
          tunnel: [w1941 w2071] -> w1398
          tunnel: [w1939 w2071] -> w1396
          tunnel: w1397 -> [w1938 _]
          tunnel: w1395 -> [w1937 _]
          tunnel: [w1936 w2071] -> w1394
          tunnel: w1393 -> [w1934 _]
          tunnel: [w1935 w2071] -> w1392
          tunnel: w1391 -> [w1933 _]
          tunnel: [w1932 w2071] -> w1390
          tunnel: w1389 -> [w1931 _]
          tunnel: [w1930 w2071] -> w1388
          tunnel: w1387 -> [w1929 _]
          tunnel: [w1923 w2071] -> w1386
          tunnel: w1385 -> [w1928 _]
          tunnel: [w1922 w2071] -> w1384
          tunnel: w1383 -> [w1927 _]
          tunnel: [w1921 w2071] -> w1382
          tunnel: w1381 -> [w1926 _]
          tunnel: [w1920 w2071] -> w1380
          tunnel: w1379 -> [w1925 _]
          tunnel: [w1919 w2071] -> w1378
          tunnel: w1377 -> [w1924 _]
          tunnel: [w1918 w2071] -> w1376
          tunnel: w1375 -> [w1916 _]
          tunnel: [w1915 w2071] -> w1374
          tunnel: w1373 -> [w1914 _]
          tunnel: [w1913 w2071] -> w1372
          tunnel: w1371 -> [w1911 _]
          tunnel: [w1912 w2071] -> w1370
          tunnel: w1369 -> [w1910 _]
          tunnel: [w1909 w2071] -> w1368
          tunnel: w1367 -> [w1908 _]
          tunnel: [w1907 w2071] -> w1366
          tunnel: w1365 -> [w1906 _]
          tunnel: [w1905 w2071] -> w1364
          tunnel: w1363 -> [w1904 _]
          tunnel: [w1903 w2071] -> w1362
          tunnel: w1361 -> [w1902 _]
          tunnel: [w1901 w2071] -> w1360
          tunnel: w1359 -> [w1900 _]
          tunnel: [w1899 w2071] -> w1358
          tunnel: [w1897 w2071] -> w1356
          tunnel: w1357 -> [w1898 _]
          tunnel: w1355 -> [w1896 _]
          tunnel: [w1895 w2071] -> w1354
          tunnel: w1353 -> [w1894 _]
          tunnel: [w1893 w2071] -> w1352
          tunnel: w1351 -> [w1992 _]
          tunnel: [w1992 w2074] -> w1350
          tunnel: w1349 -> [w2018 _]
          tunnel: [w2018 w2073] -> w1348
          tunnel: w1347 -> [w2017 _]
          tunnel: [w2017 w2075] -> w1346
          tunnel: w1289 -> [_ w2074]
          tunnel: w1288 -> [_ w2073]
          tunnel: [w2016 w2071] -> w1229
          tunnel: w1230 -> [w2016 _]
          tunnel: [w2015 w2071] -> w1227
          tunnel: w1228 -> [w2015 _]
          tunnel: w1226 -> [w2014 _]
          tunnel: [w2014 w2071] -> w1225
          tunnel: [w2013 w2071] -> w1223
          tunnel: w1224 -> [w2013 _]
          tunnel: w1222 -> [w2012 _]
          tunnel: [w2012 w2071] -> w1221
          tunnel: [w2011 w2071] -> w1214
          tunnel: w1215 -> [w2011 _]
          tunnel: w1210 -> [w2010 _]
          tunnel: [w2010 w2071] -> w1209
          tunnel: w1208 -> [w2009 _]
          tunnel: [w2009 w2071] -> w1207
          tunnel: w1206 -> [w2008 _]
          tunnel: [w2008 w2071] -> w1205
          tunnel: w1204 -> [w2007 _]
          tunnel: [w2007 w2071] -> w1203
          tunnel: w1202 -> [w2006 _]
          tunnel: [w2006 w2071] -> w1201
          tunnel: w1200 -> [w2005 _]
          tunnel: [w2005 w2071] -> w1199
          tunnel: w1191 -> [w2004 _]
          tunnel: [w2004 w2071] -> w1190
          tunnel: [w2003 w2071] -> w1189
          tunnel: w1188 -> [w2003 _]
          tunnel: w1187 -> [w2002 _]
          tunnel: [w2002 w2071] -> w1186
          tunnel: [w2001 w2071] -> w1184
          tunnel: w1185 -> [w2001 _]
          tunnel: [w2000 w2071] -> w1182
          tunnel: w1183 -> [w2000 _]
          tunnel: [w1999 w2071] -> w1180
          tunnel: w1181 -> [w1999 _]
          tunnel: w1179 -> [w1998 _]
          tunnel: [w1998 w2071] -> w1178
          tunnel: w1170 -> [w1997 _]
          tunnel: [w1997 w2071] -> w1169
          tunnel: [w1996 w2071] -> w1167
          tunnel: w1168 -> [w1996 _]
          tunnel: w1166 -> [w1995 _]
          tunnel: [w1995 w2071] -> w1165
          tunnel: w1164 -> [w1994 _]
          tunnel: [w1994 w2071] -> w1163
          tunnel: w1162 -> [w1993 _]
          tunnel: [w1993 w2071] -> w1161
          tunnel: w1098 -> [w1891 w2071]
          frame False {
            n507 = case shown="False" "Clear_L1" {
              tunnel: [w2069 w2070] -> w1991
              tunnel: w1990 -> [w2069 _]
              tunnel: [w2068 w2070] -> w1989
              tunnel: w1988 -> [w2068 _]
              tunnel: [w2067 w2070] -> w1987
              tunnel: w1986 -> [w2067 _]
              tunnel: [w2066 w2070] -> w1985
              tunnel: w1984 -> [w2066 _]
              tunnel: [w2065 w2070] -> w1983
              tunnel: w1982 -> [w2065 _]
              tunnel: [w2064 w2070] -> w1981
              tunnel: w1980 -> [w2064 _]
              tunnel: [w2063 w2070] -> w1979
              tunnel: w1978 -> [w2063 _]
              tunnel: [w2062 w2070] -> w1977
              tunnel: w1976 -> [w2062 _]
              tunnel: [w2061 w2070] -> w1975
              tunnel: w1974 -> [w2061 _]
              tunnel: [w2060 w2070] -> w1973
              tunnel: w1972 -> [w2060 _]
              tunnel: [w2059 w2070] -> w1970
              tunnel: w1971 -> [w2059 _]
              tunnel: w1969 -> [w2058 _]
              tunnel: [w2058 w2070] -> w1968
              tunnel: w1891 -> [_ w2070]
              frame False {
              }
              frame True {
              }
            }
            n508 = case shown="False" "Clear_L2" {
              tunnel: w1966 -> [w2056 _]
              tunnel: [w2056 w2057] -> w1965
              tunnel: [w2055 w2057] -> w1964
              tunnel: w1963 -> [w2055 _]
              tunnel: [w2054 w2057] -> w1961
              tunnel: w1962 -> [w2054 _]
              tunnel: [w2053 w2057] -> w1959
              tunnel: w1960 -> [w2053 _]
              tunnel: [w2052 w2057] -> w1958
              tunnel: w1957 -> [w2052 _]
              tunnel: [w2051 w2057] -> w1955
              tunnel: w1956 -> [w2051 _]
              tunnel: [w2050 w2057] -> w1954
              tunnel: w1953 -> [w2050 _]
              tunnel: [w2049 w2057] -> w1952
              tunnel: w1951 -> [w2049 _]
              tunnel: [w2048 w2057] -> w1950
              tunnel: w1949 -> [w2048 _]
              tunnel: [w2047 w2057] -> w1948
              tunnel: w1947 -> [w2047 _]
              tunnel: [w2046 w2057] -> w1945
              tunnel: w1946 -> [w2046 _]
              tunnel: [w2045 w2057] -> w1944
              tunnel: w1943 -> [w2045 _]
              tunnel: w1891 -> [_ w2057]
              frame False {
              }
              frame True {
              }
            }
            n509 = case shown="False" "Clear_L3" {
              tunnel: [w2043 w2044] -> w1941
              tunnel: w1940 -> [w2043 _]
              tunnel: [w2042 w2044] -> w1939
              tunnel: w1938 -> [w2042 _]
              tunnel: [w2041 w2044] -> w1936
              tunnel: w1937 -> [w2041 _]
              tunnel: [w2040 w2044] -> w1935
              tunnel: w1934 -> [w2040 _]
              tunnel: w1933 -> [w2039 _]
              tunnel: [w2039 w2044] -> w1932
              tunnel: w1931 -> [w2038 _]
              tunnel: [w2038 w2044] -> w1930
              tunnel: [w2037 w2044] -> w1923
              tunnel: w1929 -> [w2037 _]
              tunnel: [w2036 w2044] -> w1922
              tunnel: w1928 -> [w2036 _]
              tunnel: w1927 -> [w2035 _]
              tunnel: [w2035 w2044] -> w1921
              tunnel: [w2034 w2044] -> w1920
              tunnel: w1926 -> [w2034 _]
              tunnel: w1925 -> [w2033 _]
              tunnel: [w2033 w2044] -> w1919
              tunnel: w1924 -> [w2032 _]
              tunnel: [w2032 w2044] -> w1918
              tunnel: w1891 -> [_ w2044]
              frame False {
              }
              frame True {
              }
            }
            n510 = case shown="False" "Clear_L4" {
              tunnel: [w2030 w2031] -> w1915
              tunnel: w1916 -> [w2030 _]
              tunnel: w1914 -> [w2029 _]
              tunnel: [w2029 w2031] -> w1913
              tunnel: [w2028 w2031] -> w1912
              tunnel: w1911 -> [w2028 _]
              tunnel: [w2027 w2031] -> w1909
              tunnel: w1910 -> [w2027 _]
              tunnel: w1908 -> [w2026 _]
              tunnel: [w2026 w2031] -> w1907
              tunnel: w1906 -> [w2025 _]
              tunnel: [w2025 w2031] -> w1905
              tunnel: [w2024 w2031] -> w1903
              tunnel: w1904 -> [w2024 _]
              tunnel: w1902 -> [w2023 _]
              tunnel: [w2023 w2031] -> w1901
              tunnel: w1900 -> [w2022 _]
              tunnel: [w2022 w2031] -> w1899
              tunnel: w1898 -> [w2021 _]
              tunnel: [w2021 w2031] -> w1897
              tunnel: w1896 -> [w2020 _]
              tunnel: [w2020 w2031] -> w1895
              tunnel: w1894 -> [w2019 _]
              tunnel: [w2019 w2031] -> w1893
              tunnel: w1891 -> [_ w2031]
              frame False {
              }
              frame True {
              }
            }
          }
          frame True {
            n511 = Get Date/Time In Seconds() -> (seconds since 1Jan1904=w2072:timestamp)
            n512 = Build Array(w2072) -> (w2075:timestamp[])
          }
        }
        n513 = Index Array(array=w588) -> (element #1=w1079:bool, element #2=w1080:bool, element #3=w1084:bool, element #4=w1081:bool, element #5=w1082:bool, element #6=w1083:bool)  [unwired: 6 in]
        n514 = Index Array(array=w290) -> (element #1=w304:bool, element #2=w303:bool, element #3=w299:bool, element #4=w302:bool, element #5=w301:bool, element #6=w300:bool)  [unwired: 6 in]
        n515 = Array Subset(array=w944, index=w750, length=w751) -> (w877:dbl[])
        n516 = call "Channel_plots.vi"("Current time"=w589, "In Channels"=w876, "Input Channels"=w877) -> ("output graph"=→"L1 (St-2)  2":T2, "out Ch 1"=w858:dbl[], "out Ch 6"=w873:dbl[], "out Ch 2"=w860:dbl[], "out Ch 3"=w862:dbl[], "out Ch 4"=w864:dbl[], "out Ch 5"=w866:dbl[])
        n517 = call "Channel_plots.vi"("Current time"=w589, "In Channels"=w706, "Input Channels"=w877) -> ("output graph"=→"L1 (St-2) -I 2":T2, "out Ch 1"=w774:dbl[], "out Ch 6"=w784:dbl[], "out Ch 2"=w776:dbl[], "out Ch 3"=w778:dbl[], "out Ch 4"=w780:dbl[], "out Ch 5"=w782:dbl[])
        n518 = Array Subset(array=w944, index=w751) -> (w937:dbl[])  [unwired: 1 in]
        n519 = call "Channel_plots.vi"("Current time"=w589, "In Channels"=w896, "Input Channels"=w937) -> ("output graph"=→"L2 (St-1) 2":T2, "out Ch 1"=w878:dbl[], "out Ch 6"=w888:dbl[], "out Ch 2"=w880:dbl[], "out Ch 3"=w882:dbl[], "out Ch 4"=w884:dbl[], "out Ch 5"=w886:dbl[])
        n520 = call "Channel_plots.vi"("Current time"=w589, "In Channels"=w714, "Input Channels"=w937) -> ("output graph"=→"L2 (St-1) -I 2":T2, "out Ch 1"=w798:dbl[], "out Ch 6"=w808:dbl[], "out Ch 2"=w800:dbl[], "out Ch 3"=w802:dbl[], "out Ch 4"=w804:dbl[], "out Ch 5"=w806:dbl[])
        n521 = Array Subset(array=w945, index=w750, length=w751) -> (w936:dbl[])
        n522 = call "Channel_plots.vi"("Current time"=w589, "In Channels"=w917, "Input Channels"=w936) -> ("output graph"=→"L3 (Eta-2 ) 2":T2, "out Ch 1"=w897:dbl[], "out Ch 6"=w907:dbl[], "out Ch 2"=w900:dbl[], "out Ch 3"=w901:dbl[], "out Ch 4"=w903:dbl[], "out Ch 5"=w905:dbl[])
        n523 = call "Channel_plots.vi"("Current time"=w589, "In Channels"=w722, "Input Channels"=w936) -> ("output graph"=→"L3 (Eta-2) -I 2":T2, "out Ch 1"=w822:dbl[], "out Ch 6"=w832:dbl[], "out Ch 2"=w824:dbl[], "out Ch 3"=w826:dbl[], "out Ch 4"=w828:dbl[], "out Ch 5"=w830:dbl[])
        n524 = Array Subset(array=w945, index=w751) -> (w935:dbl[])  [unwired: 1 in]
        n525 = call "Channel_plots.vi"("Current time"=w589, "In Channels"=w934, "Input Channels"=w935) -> ("output graph"=→"L4 (Eta-1) 2":T2, "out Ch 1"=w909:dbl[], "out Ch 6"=w926:dbl[], "out Ch 2"=w918:dbl[], "out Ch 3"=w920:dbl[], "out Ch 4"=w922:dbl[], "out Ch 5"=w924:dbl[])
        n526 = call "Channel_plots.vi"("Current time"=w589, "In Channels"=w724, "Input Channels"=w935) -> ("output graph"=→"L4 (Eta-1) -I 2":T2, "out Ch 1"=w846:dbl[], "out Ch 6"=w856:dbl[], "out Ch 2"=w848:dbl[], "out Ch 3"=w850:dbl[], "out Ch 4"=w852:dbl[], "out Ch 5"=w854:dbl[])
        n527 = Array Subset(array=w942, index=w753, length=w752) -> (w758:dbl[])
        n528 = call "Channel_plots.vi"("Current time"=w589, "In Channels"=w699, "Input Channels"=w758) -> ("output graph"=→"L1 (St-2) -V 2":T2, "out Ch 1"=w762:dbl[], "out Ch 6"=w772:dbl[], "out Ch 2"=w764:dbl[], "out Ch 3"=w766:dbl[], "out Ch 4"=w768:dbl[], "out Ch 5"=w770:dbl[])
        n529 = Array Subset(array=w942, index=w752) -> (w759:dbl[])  [unwired: 1 in]
        n530 = call "Channel_plots.vi"("Current time"=w589, "In Channels"=w707, "Input Channels"=w759) -> ("output graph"=→"L2 (St-1) -V 2":T2, "out Ch 1"=w786:dbl[], "out Ch 6"=w796:dbl[], "out Ch 2"=w788:dbl[], "out Ch 3"=w790:dbl[], "out Ch 4"=w792:dbl[], "out Ch 5"=w794:dbl[])
        n531 = Array Subset(array=w943, index=w753, length=w752) -> (w760:dbl[])
        n532 = call "Channel_plots.vi"("Current time"=w589, "In Channels"=w721, "Input Channels"=w760) -> ("output graph"=→"L3 (Eta-2) -V 2":T2, "out Ch 1"=w810:dbl[], "out Ch 6"=w820:dbl[], "out Ch 2"=w812:dbl[], "out Ch 3"=w814:dbl[], "out Ch 4"=w816:dbl[], "out Ch 5"=w818:dbl[])
        n533 = Array Subset(array=w943, index=w752) -> (w761:dbl[])  [unwired: 1 in]
        n534 = call "Channel_plots.vi"("Current time"=w589, "In Channels"=w723, "Input Channels"=w761) -> ("output graph"=→"L4 (Eta-1) -V 2":T2, "out Ch 1"=w834:dbl[], "out Ch 6"=w844:dbl[], "out Ch 2"=w836:dbl[], "out Ch 3"=w838:dbl[], "out Ch 4"=w840:dbl[], "out Ch 5"=w842:dbl[])
        n535 = case shown="False" w681 {
          tunnel: w762 -> [w1726 _]
          tunnel: [w1727 w1804] -> w763
          tunnel: [w1725 w1804] -> w765
          tunnel: w764 -> [w1724 _]
          tunnel: [w1723 w1804] -> w767
          tunnel: w766 -> [w1722 _]
          tunnel: [w1721 w1804] -> w769
          tunnel: w768 -> [w1720 _]
          tunnel: [w1719 w1804] -> w771
          tunnel: w770 -> [w1718 _]
          tunnel: [w1717 w1804] -> w773
          tunnel: w772 -> [w1716 _]
          tunnel: w774 -> [w1714 _]
          tunnel: [w1715 w1804] -> w775
          tunnel: w776 -> [w1712 _]
          tunnel: [w1713 w1804] -> w777
          tunnel: w778 -> [w1710 _]
          tunnel: [w1711 w1804] -> w779
          tunnel: w780 -> [w1708 _]
          tunnel: [w1709 w1804] -> w781
          tunnel: w782 -> [w1707 _]
          tunnel: [w1706 w1804] -> w783
          tunnel: w784 -> [w1705 _]
          tunnel: [w1704 w1804] -> w785
          tunnel: w786 -> [w1703 _]
          tunnel: [w1702 w1804] -> w787
          tunnel: w788 -> [w1700 _]
          tunnel: [w1701 w1804] -> w789
          tunnel: w790 -> [w1699 _]
          tunnel: [w1698 w1804] -> w791
          tunnel: w792 -> [w1697 _]
          tunnel: [w1696 w1804] -> w793
          tunnel: [w1695 w1804] -> w795
          tunnel: w794 -> [w1694 _]
          tunnel: [w1692 w1804] -> w797
          tunnel: w796 -> [w1693 _]
          tunnel: [w1691 w1804] -> w799
          tunnel: w798 -> [w1690 _]
          tunnel: [w1689 w1804] -> w801
          tunnel: w800 -> [w1688 _]
          tunnel: w802 -> [w1686 _]
          tunnel: [w1687 w1804] -> w803
          tunnel: [w1685 w1804] -> w805
          tunnel: w804 -> [w1684 _]
          tunnel: w806 -> [w1683 _]
          tunnel: [w1682 w1804] -> w807
          tunnel: w808 -> [w1680 _]
          tunnel: [w1681 w1804] -> w809
          tunnel: w810 -> [w1678 _]
          tunnel: [w1679 w1804] -> w811
          tunnel: [w1677 w1804] -> w813
          tunnel: w812 -> [w1676 _]
          tunnel: w814 -> [w1675 _]
          tunnel: [w1674 w1804] -> w815
          tunnel: w816 -> [w1672 _]
          tunnel: [w1673 w1804] -> w817
          tunnel: w818 -> [w1671 _]
          tunnel: [w1670 w1804] -> w819
          tunnel: w820 -> [w1669 _]
          tunnel: [w1668 w1804] -> w821
          tunnel: w822 -> [w1667 _]
          tunnel: [w1661 w1804] -> w823
          tunnel: w824 -> [w1666 _]
          tunnel: [w1660 w1804] -> w825
          tunnel: w826 -> [w1665 _]
          tunnel: [w1659 w1804] -> w827
          tunnel: w828 -> [w1664 _]
          tunnel: [w1658 w1804] -> w829
          tunnel: w830 -> [w1663 _]
          tunnel: [w1657 w1804] -> w831
          tunnel: w832 -> [w1662 _]
          tunnel: [w1656 w1804] -> w833
          tunnel: w834 -> [w1655 _]
          tunnel: [w1654 w1804] -> w835
          tunnel: w836 -> [w1653 _]
          tunnel: [w1652 w1804] -> w837
          tunnel: w838 -> [w1650 _]
          tunnel: [w1651 w1804] -> w839
          tunnel: w840 -> [w1649 _]
          tunnel: [w1648 w1804] -> w841
          tunnel: w842 -> [w1647 _]
          tunnel: [w1646 w1804] -> w843
          tunnel: w844 -> [w1645 _]
          tunnel: [w1644 w1804] -> w845
          tunnel: w846 -> [w1643 _]
          tunnel: [w1642 w1804] -> w847
          tunnel: w848 -> [w1641 _]
          tunnel: [w1640 w1804] -> w849
          tunnel: w850 -> [w1639 _]
          tunnel: [w1638 w1804] -> w851
          tunnel: [w1636 w1804] -> w853
          tunnel: w852 -> [w1637 _]
          tunnel: w854 -> [w1635 _]
          tunnel: [w1634 w1804] -> w855
          tunnel: w856 -> [w1633 _]
          tunnel: [w1632 w1804] -> w857
          tunnel: [w1751 w1804] -> w859
          tunnel: w858 -> [w1751 _]
          tunnel: [w1750 w1804] -> w861
          tunnel: w860 -> [w1750 _]
          tunnel: w862 -> [w1749 _]
          tunnel: [w1749 w1804] -> w863
          tunnel: [w1748 w1804] -> w865
          tunnel: w864 -> [w1748 _]
          tunnel: w866 -> [w1747 _]
          tunnel: [w1747 w1804] -> w867
          tunnel: [w1746 w1804] -> w874
          tunnel: w873 -> [w1746 _]
          tunnel: w878 -> [w1745 _]
          tunnel: [w1745 w1804] -> w879
          tunnel: w880 -> [w1744 _]
          tunnel: [w1744 w1804] -> w881
          tunnel: w882 -> [w1743 _]
          tunnel: [w1743 w1804] -> w883
          tunnel: w884 -> [w1742 _]
          tunnel: [w1742 w1804] -> w885
          tunnel: w886 -> [w1741 _]
          tunnel: [w1741 w1804] -> w887
          tunnel: w888 -> [w1740 _]
          tunnel: [w1740 w1804] -> w889
          tunnel: w897 -> [w1739 _]
          tunnel: [w1739 w1804] -> w898
          tunnel: [w1738 w1804] -> w899
          tunnel: w900 -> [w1738 _]
          tunnel: w901 -> [w1737 _]
          tunnel: [w1737 w1804] -> w902
          tunnel: [w1736 w1804] -> w904
          tunnel: w903 -> [w1736 _]
          tunnel: [w1735 w1804] -> w906
          tunnel: w905 -> [w1735 _]
          tunnel: [w1734 w1804] -> w908
          tunnel: w907 -> [w1734 _]
          tunnel: w909 -> [w1733 _]
          tunnel: [w1733 w1804] -> w910
          tunnel: w918 -> [w1732 _]
          tunnel: [w1732 w1804] -> w919
          tunnel: [w1731 w1804] -> w921
          tunnel: w920 -> [w1731 _]
          tunnel: w922 -> [w1730 _]
          tunnel: [w1730 w1804] -> w923
          tunnel: w924 -> [w1729 _]
          tunnel: [w1729 w1804] -> w925
          tunnel: w926 -> [w1728 _]
          tunnel: [w1728 w1804] -> w927
          tunnel: w946 -> [w1631 w1804]
          frame False {
            n536 = case shown="False" "Clear_L1 2" {
              tunnel: [w1802 w1803] -> w1727
              tunnel: w1726 -> [w1802 _]
              tunnel: [w1801 w1803] -> w1725
              tunnel: w1724 -> [w1801 _]
              tunnel: [w1800 w1803] -> w1723
              tunnel: w1722 -> [w1800 _]
              tunnel: [w1799 w1803] -> w1721
              tunnel: w1720 -> [w1799 _]
              tunnel: [w1798 w1803] -> w1719
              tunnel: w1718 -> [w1798 _]
              tunnel: [w1797 w1803] -> w1717
              tunnel: w1716 -> [w1797 _]
              tunnel: [w1796 w1803] -> w1715
              tunnel: w1714 -> [w1796 _]
              tunnel: [w1795 w1803] -> w1713
              tunnel: w1712 -> [w1795 _]
              tunnel: [w1794 w1803] -> w1711
              tunnel: w1710 -> [w1794 _]
              tunnel: [w1793 w1803] -> w1709
              tunnel: w1708 -> [w1793 _]
              tunnel: [w1792 w1803] -> w1706
              tunnel: w1707 -> [w1792 _]
              tunnel: w1705 -> [w1791 _]
              tunnel: [w1791 w1803] -> w1704
              tunnel: w1631 -> [_ w1803]
              frame False {
              }
              frame True {
              }
            }
            n537 = case shown="False" "Clear_L2 2" {
              tunnel: w1703 -> [w1789 _]
              tunnel: [w1789 w1790] -> w1702
              tunnel: [w1788 w1790] -> w1701
              tunnel: w1700 -> [w1788 _]
              tunnel: [w1787 w1790] -> w1698
              tunnel: w1699 -> [w1787 _]
              tunnel: [w1786 w1790] -> w1696
              tunnel: w1697 -> [w1786 _]
              tunnel: [w1785 w1790] -> w1695
              tunnel: w1694 -> [w1785 _]
              tunnel: [w1784 w1790] -> w1692
              tunnel: w1693 -> [w1784 _]
              tunnel: [w1783 w1790] -> w1691
              tunnel: w1690 -> [w1783 _]
              tunnel: [w1782 w1790] -> w1689
              tunnel: w1688 -> [w1782 _]
              tunnel: [w1781 w1790] -> w1687
              tunnel: w1686 -> [w1781 _]
              tunnel: [w1780 w1790] -> w1685
              tunnel: w1684 -> [w1780 _]
              tunnel: [w1779 w1790] -> w1682
              tunnel: w1683 -> [w1779 _]
              tunnel: [w1778 w1790] -> w1681
              tunnel: w1680 -> [w1778 _]
              tunnel: w1631 -> [_ w1790]
              frame False {
              }
              frame True {
              }
            }
            n538 = case shown="False" "Clear_L3 2" {
              tunnel: [w1776 w1777] -> w1679
              tunnel: w1678 -> [w1776 _]
              tunnel: [w1775 w1777] -> w1677
              tunnel: w1676 -> [w1775 _]
              tunnel: [w1774 w1777] -> w1674
              tunnel: w1675 -> [w1774 _]
              tunnel: [w1773 w1777] -> w1673
              tunnel: w1672 -> [w1773 _]
              tunnel: w1671 -> [w1772 _]
              tunnel: [w1772 w1777] -> w1670
              tunnel: w1669 -> [w1771 _]
              tunnel: [w1771 w1777] -> w1668
              tunnel: [w1770 w1777] -> w1661
              tunnel: w1667 -> [w1770 _]
              tunnel: [w1769 w1777] -> w1660
              tunnel: w1666 -> [w1769 _]
              tunnel: w1665 -> [w1768 _]
              tunnel: [w1768 w1777] -> w1659
              tunnel: [w1767 w1777] -> w1658
              tunnel: w1664 -> [w1767 _]
              tunnel: w1663 -> [w1766 _]
              tunnel: [w1766 w1777] -> w1657
              tunnel: w1662 -> [w1765 _]
              tunnel: [w1765 w1777] -> w1656
              tunnel: w1631 -> [_ w1777]
              frame False {
              }
              frame True {
              }
            }
            n539 = case shown="False" "Clear_L4 2" {
              tunnel: [w1763 w1764] -> w1654
              tunnel: w1655 -> [w1763 _]
              tunnel: w1653 -> [w1762 _]
              tunnel: [w1762 w1764] -> w1652
              tunnel: [w1761 w1764] -> w1651
              tunnel: w1650 -> [w1761 _]
              tunnel: [w1760 w1764] -> w1648
              tunnel: w1649 -> [w1760 _]
              tunnel: w1647 -> [w1759 _]
              tunnel: [w1759 w1764] -> w1646
              tunnel: w1645 -> [w1758 _]
              tunnel: [w1758 w1764] -> w1644
              tunnel: [w1757 w1764] -> w1642
              tunnel: w1643 -> [w1757 _]
              tunnel: w1641 -> [w1756 _]
              tunnel: [w1756 w1764] -> w1640
              tunnel: w1639 -> [w1755 _]
              tunnel: [w1755 w1764] -> w1638
              tunnel: w1637 -> [w1754 _]
              tunnel: [w1754 w1764] -> w1636
              tunnel: w1635 -> [w1753 _]
              tunnel: [w1753 w1764] -> w1634
              tunnel: w1633 -> [w1752 _]
              tunnel: [w1752 w1764] -> w1632
              tunnel: w1631 -> [_ w1764]
              frame False {
              }
              frame True {
              }
            }
          }
          frame True {
          }
        }
        n540 = Not(x=w1079) -> (.not. x?=→"8-R_Gr_L2":bool)
        n541 = Not(x=w1080) -> (.not. x?=→"8-L_Gr_L2":bool)
        n542 = Not(x=w1084) -> (.not. x?=→"7-R_Gr_L2":bool)
        n543 = Not(x=w1081) -> (.not. x?=→"7-L_Gr_L2":bool)
        n544 = Not(x=w1082) -> (.not. x?=→"6-R_Gr_L2":bool)
        n545 = Not(x=w1083) -> (.not. x?=→"6-L_Gr_L2":bool)
        n546 = Not(x=w304) -> (.not. x?=→"8-R_Gr_L2 2":bool)
        n547 = Not(x=w303) -> (.not. x?=→"8-L_Gr_L2 2":bool)
        n548 = Not(x=w299) -> (.not. x?=→"7-R_Gr_L2 2":bool)
        n549 = Not(x=w302) -> (.not. x?=→"7-L_Gr_L2 2":bool)
        n550 = Not(x=w301) -> (.not. x?=→"6-R_Gr_L2 2":bool)
        n551 = Not(x=w300) -> (.not. x?=→"6-L_Gr_L2 2":bool)
        n552 = Build Array(w1211, w1459) -> (w1463:dbl[][])
        n553 = Build Array(w1151, w1458) -> (w1462:dbl[][])
        n554 = Build Array(w1152, w1457) -> (w1461:dbl[][])
        n555 = Build Array(w1153, w1456) -> (w1460:dbl[][])
        n556 = Build Array(w877, w758) -> (w754:dbl[][])
        n557 = Build Array(w937, w759) -> (w755:dbl[][])
        n558 = Build Array(w936, w760) -> (w756:dbl[][])
        n559 = Build Array(w935, w761) -> (w757:dbl[][])
        n560 = Transpose 2D Array(2D array=w1463) -> (transposed array=w1147:dbl[][])
        n561 = Transpose 2D Array(2D array=w1462) -> (transposed array=w1146:dbl[][])
        n562 = Transpose 2D Array(2D array=w1461) -> (transposed array=w1145:dbl[][])
        n563 = Transpose 2D Array(2D array=w1460) -> (transposed array=w1144:dbl[][])
        n564 = call "Save_file.vi"("Save path"=w1528, "Presure"=w1526, "current time"=w442, "Save"=w1527, "Temperature"=w1525, "M L1 (eta1)"=w1147, "M L2 (eta2)"=w1146, "M L3 (Stereo 1)"=w1145, "M L4 (Stereo 2)"=w1144) -> ()
        n565 = Transpose 2D Array(2D array=w754) -> (transposed array=w456:dbl[][])
        n566 = Transpose 2D Array(2D array=w755) -> (transposed array=w455:dbl[][])
        n567 = Transpose 2D Array(2D array=w756) -> (transposed array=w454:dbl[][])
        n568 = Transpose 2D Array(2D array=w757) -> (transposed array=w453:dbl[][])
        n569 = call "Save_file.vi"("Save path"=w650, "Presure"=w697, "current time"=w442, "Save"=w649, "Temperature"=w698, "M L1 (eta1)"=w456, "M L2 (eta2)"=w455, "M L3 (Stereo 1)"=w454, "M L4 (Stereo 2)"=w453) -> ()
        n570 = Index Array(array=w587) -> (element #1=w1067:bool, element #2=w1072:bool, element #3=w1068:bool, element #4=w1071:bool, element #5=w1070:bool, element #6=w1069:bool)  [unwired: 6 in]
        n571 = Index Array(array=w289) -> (element #1=w310:bool, element #2=w305:bool, element #3=w309:bool, element #4=w306:bool, element #5=w307:bool, element #6=w308:bool)  [unwired: 6 in]
        n572 = Index Array(array=w455, index (row) #1=0 ("index (row)"), index (col) #1=w633, index (row) #2=1 ("index (row)"), index (col) #2=w633, index (row) #3=2 ("index (row)"), index (col) #3=w633, index (row) #4=3 ("index (row)"), index (col) #4=w633, index (row) #5=4 ("index (row)"), index (col) #5=w633, index (row) #6=5 ("index (row)"), index (col) #6=w633) -> (element #1=→"L2_S8-1R_ind 2":dbl, element #2=→"L2_S8-1L_ind 2":dbl, element #3=→"L2_S7-1R_ind 2":dbl, element #4=→"L2_S7-1L_ind 2":dbl, element #5=→"L2_S6-1R_ind 2":dbl, element #6=→"L2_S6-1L_ind 2":dbl)
        n573 = Index Array(array=w453, index (row) #1=0 ("index (row)"), index (col) #1=w605, index (row) #2=1 ("index (row)"), index (col) #2=w605, index (row) #3=2 ("index (row)"), index (col) #3=w605, index (row) #4=3 ("index (row)"), index (col) #4=w605, index (row) #5=4 ("index (row)"), index (col) #5=w605, index (row) #6=5 ("index (row)"), index (col) #6=w605) -> (element #1=→"L4_E8-1R_ind 2":dbl, element #2=→"L4_E8-1L_ind 2":dbl, element #3=→"L4_E7-1R_ind 2":dbl, element #4=→"L4_E7-1L_ind 2":dbl, element #5=→"L4_E6-1R_ind 2":dbl, element #6=→"L4_E6-1L_ind 2":dbl)
        n574 = Not(x=w1067) -> (.not. x?=→"8-R_Gr_L3":bool)
        n575 = Not(x=w1072) -> (.not. x?=→"8-L_Gr_L3":bool)
        n576 = Not(x=w1068) -> (.not. x?=→"7-R_Gr_L3":bool)
        n577 = Not(x=w1071) -> (.not. x?=→"7-L_Gr_L3":bool)
        n578 = Not(x=w1070) -> (.not. x?=→"6-R_Gr_L3":bool)
        n579 = Not(x=w1069) -> (.not. x?=→"6-L_Gr_L3":bool)
        n580 = Not(x=w310) -> (.not. x?=→"8-R_Gr_L3 2":bool)
        n581 = Not(x=w305) -> (.not. x?=→"8-L_Gr_L3 2":bool)
        n582 = Not(x=w309) -> (.not. x?=→"7-R_Gr_L3 2":bool)
        n583 = Not(x=w306) -> (.not. x?=→"7-L_Gr_L3 2":bool)
        n584 = Not(x=w307) -> (.not. x?=→"6-R_Gr_L3 2":bool)
        n585 = Not(x=w308) -> (.not. x?=→"6-L_Gr_L3 2":bool)
        n586 = property on="L2 (St-1) -V 2" class="XYGraph (strict)"("BG Color"="Graphs bachground Color") -> ()  [unwired: 2 in, 2 out]
        n587 = property on="L2 (St-1) -I 2" class="XYGraph (strict)"("BG Color"="Graphs bachground Color") -> ()  [unwired: 2 in, 2 out]
        n588 = property on="L2 (St-1) -V" class="XYGraph (strict)"("BG Color"="Graphs bachground Color") -> ()  [unwired: 2 in, 2 out]
        n589 = property on="L2 (St-1) -I" class="XYGraph (strict)"("BG Color"="Graphs bachground Color") -> ()  [unwired: 2 in, 2 out]
        n590 = property on="L1 (St-2)  2" class="XYGraph (strict)"("YScale.Mapping Mode"=w659) -> ()  [unwired: 2 in, 2 out]
        n591 = property on="L2 (St-1) 2" class="XYGraph (strict)"("YScale.Mapping Mode"=w659) -> ()  [unwired: 2 in, 2 out]
        n592 = property on="L3 (Eta-2 ) 2" class="XYGraph (strict)"("YScale.Mapping Mode"=w659) -> ()  [unwired: 2 in, 2 out]
        n593 = property on="L4 (Eta-1) 2" class="XYGraph (strict)"("YScale.Mapping Mode"=w659) -> ()  [unwired: 2 in, 2 out]
        n594 = Bundle("Value"=w168, "Value"=w169, "Value"=w170, "Value"=w171, "Value"=w172, "Value"=w173, "Value"=w174, "Value"=w175, "Value"=w176, "Value"=w177, "Value"=w178, "Value"=w179, "Value"=w162) -> (w180:T8)  [unwired: 1 in]
        n595 = Index Array(array=w456, index (row) #1=0 ("index (row)"), index (col) #1=w516, index (row) #2=1 ("index (row)"), index (col) #2=w516, index (row) #3=2 ("index (row)"), index (col) #3=w516, index (row) #4=3 ("index (row)"), index (col) #4=w516, index (row) #5=4 ("index (row)"), index (col) #5=w516, index (row) #6=5 ("index (row)"), index (col) #6=w516, index (row) #7=0 ("index (row)"), index (col) #7=w510, index (row) #8=1 ("index (row)"), index (col) #8=w510, index (row) #9=2 ("index (row)"), index (col) #9=w510, index (row) #10=3 ("index (row)"), index (col) #10=w510, index (row) #11=4 ("index (row)"), index (col) #11=w510, index (row) #12=5 ("index (row)"), index (col) #12=w510) -> (element #1=→"S8-2R I 2":dbl, element #2=→"S8-2L I 2":dbl, element #3=→"S7-2R I 2":dbl, element #4=→"S7-2L I 2":dbl, element #5=→"S6-2R I 2":dbl, element #6=→"S6-2L I 2":dbl, element #7=→"S8-2R V 2":dbl, element #8=→"S8-2L V 2":dbl, element #9=→"S7-2R V 2":dbl, element #10=→"S7-2L V 2":dbl, element #11=→"S6-2R V 2":dbl, element #12=→"S6-2L V 2":dbl)
        n596 = Index Array(array=w455, index (row) #1=0 ("index (row)"), index (col) #1=w521, index (row) #2=1 ("index (row)"), index (col) #2=w521, index (row) #3=2 ("index (row)"), index (col) #3=w521, index (row) #4=3 ("index (row)"), index (col) #4=w521, index (row) #5=4 ("index (row)"), index (col) #5=w521, index (row) #6=5 ("index (row)"), index (col) #6=w521, index (row) #7=0 ("index (row)"), index (col) #7=w527, index (row) #8=1 ("index (row)"), index (col) #8=w527, index (row) #9=2 ("index (row)"), index (col) #9=w527, index (row) #10=3 ("index (row)"), index (col) #10=w527, index (row) #11=4 ("index (row)"), index (col) #11=w527, index (row) #12=5 ("index (row)"), index (col) #12=w527) -> (element #1=→"S8-1R I 2":dbl, element #2=→"S8-1L I 2":dbl, element #3=→"S7-1R I 2":dbl, element #4=→"S7-1L I 2":dbl, element #5=→"S6-1R I 2":dbl, element #6=→"S6-1L I 2":dbl, element #7=→"S8-1R V 2":dbl, element #8=→"S8-1L V 2":dbl, element #9=→"S7-1R V 2":dbl, element #10=→"S7-1L V 2":dbl, element #11=→"S6-1R V 2":dbl, element #12=→"S6-1L V 2":dbl)
        n597 = property on="L3 (Eta-2) -I 2" class="XYGraph (strict)"("BG Color"="Graphs bachground Color") -> ()  [unwired: 2 in, 2 out]
        n598 = property on="L3 (Eta-2) -V 2" class="XYGraph (strict)"("BG Color"="Graphs bachground Color") -> ()  [unwired: 2 in, 2 out]
        n599 = property on="L3 (Eta-2) -I" class="XYGraph (strict)"("BG Color"="Graphs bachground Color") -> ()  [unwired: 2 in, 2 out]
        n600 = property on="L3 (Eta-2) -V" class="XYGraph (strict)"("BG Color"="Graphs bachground Color") -> ()  [unwired: 2 in, 2 out]
        n601 = Multiply(x="Delay [s]", y=u32 1000) -> (x*y=w593:dbl)
        n602 = Index Array(array=w1147, index (row) #1=0 ("index (row)"), index (col) #1=w1334, index (row) #2=1 ("index (row)"), index (col) #2=w1334, index (row) #3=2 ("index (row)"), index (col) #3=w1334, index (row) #4=3 ("index (row)"), index (col) #4=w1334, index (row) #5=4 ("index (row)"), index (col) #5=w1334, index (row) #6=5 ("index (row)"), index (col) #6=w1334, index (row) #7=0 ("index (row)"), index (col) #7=w1340, index (row) #8=1 ("index (row)"), index (col) #8=w1340, index (row) #9=2 ("index (row)"), index (col) #9=w1340, index (row) #10=3 ("index (row)"), index (col) #10=w1340, index (row) #11=4 ("index (row)"), index (col) #11=w1340, index (row) #12=5 ("index (row)"), index (col) #12=w1340) -> (element #1=→"S8-2R I":dbl, element #2=→"S8-2L I":dbl, element #3=→"S7-2R I":dbl, element #4=→"S7-2L I":dbl, element #5=→"S6-2R I":dbl, element #6=→"S6-2L I":dbl, element #7=→"S8-2R V":dbl, element #8=→"S8-2L V":dbl, element #9=→"S7-2R V":dbl, element #10=→"S7-2L V":dbl, element #11=→"S6-2R V":dbl, element #12=→"S6-2L V":dbl)
        n603 = Index Array(array=w1146, index (row) #1=0 ("index (row)"), index (col) #1=w1329, index (row) #2=1 ("index (row)"), index (col) #2=w1329, index (row) #3=2 ("index (row)"), index (col) #3=w1329, index (row) #4=3 ("index (row)"), index (col) #4=w1329, index (row) #5=4 ("index (row)"), index (col) #5=w1329, index (row) #6=5 ("index (row)"), index (col) #6=w1329, index (row) #7=0 ("index (row)"), index (col) #7=w1323, index (row) #8=1 ("index (row)"), index (col) #8=w1323, index (row) #9=2 ("index (row)"), index (col) #9=w1323, index (row) #10=3 ("index (row)"), index (col) #10=w1323, index (row) #11=4 ("index (row)"), index (col) #11=w1323, index (row) #12=5 ("index (row)"), index (col) #12=w1323) -> (element #1=→"S8-1R I":dbl, element #2=→"S8-1L I":dbl, element #3=→"S7-1R I":dbl, element #4=→"S7-1L I":dbl, element #5=→"S6-1R I":dbl, element #6=→"S6-1L I":dbl, element #7=→"S8-1R V":dbl, element #8=→"S8-1L V":dbl, element #9=→"S7-1R V":dbl, element #10=→"S7-1L V":dbl, element #11=→"S6-1R V":dbl, element #12=→"S6-1L V":dbl)
        n604 = local read "E6-1L I"() -> (w959:dbl)
        n605 = local read "E6-1R I"() -> (w958:dbl)
        n606 = local read "E7-1L I"() -> (w957:dbl)
        n607 = local read "E7-1R I"() -> (w956:dbl)
        n608 = local read "E8-1L I"() -> (w955:dbl)
        n609 = local read "E8-1R I"() -> (w954:dbl)
        n610 = local read "E6-1L I"() -> (w335:dbl)
        n611 = local read "E6-1R I"() -> (w336:dbl)
        n612 = local read "E7-1L I"() -> (w337:dbl)
        n613 = local read "E7-1R I"() -> (w338:dbl)
        n614 = local read "E8-1L I"() -> (w339:dbl)
        n615 = local read "E8-1R I"() -> (w340:dbl)
        n616 = call "Config.vi"("Config_W/R"="Set configure", "Config"=w180) -> ()  [unwired: 1 out]
        n617 = Wait (ms)(milliseconds to wait=w593) -> ()  [unwired: 1 out]
        n618 = property on="L4 (Eta-1) -V 2" class="XYGraph (strict)"("BG Color"="Graphs bachground Color") -> ()  [unwired: 2 in, 2 out]
        n619 = property on="L4 (Eta-1) -I 2" class="XYGraph (strict)"("BG Color"="Graphs bachground Color") -> ()  [unwired: 2 in, 2 out]
        n620 = property on="L4 (Eta-1) -V" class="XYGraph (strict)"("BG Color"="Graphs bachground Color") -> ()  [unwired: 2 in, 2 out]
        n621 = property on="L4 (Eta-1) -I" class="XYGraph (strict)"("BG Color"="Graphs bachground Color") -> ()  [unwired: 2 in, 2 out]
        n622 = Index Array(array=w586) -> (element #1=w1061:bool, element #2=w1056:bool, element #3=w1060:bool, element #4=w1057:bool, element #5=w1058:bool, element #6=w1059:bool)  [unwired: 6 in]
        n623 = Index Array(array=w288) -> (element #1=w311:bool, element #2=w316:bool, element #3=w312:bool, element #4=w315:bool, element #5=w314:bool, element #6=w313:bool)  [unwired: 6 in]
        n624 = call "Level.vi"("Y_Lev_max"=w951, "IN"=w959, "G_Lev_max"=w953) -> ("R"=→"6-L_R_L4":bool, "Y"=→"6-L_Y_L4":bool, "G"=→"6-L_G_L4":bool)
        n625 = call "Level.vi"("Y_Lev_max"=w951, "IN"=w958, "G_Lev_max"=w953) -> ("R"=→"6-R_R_L4":bool, "Y"=→"6-R_Y_L4":bool, "G"=→"6-R_G_L4":bool)
        n626 = call "Level.vi"("Y_Lev_max"=w951, "IN"=w957, "G_Lev_max"=w953) -> ("R"=→"7-L_R_L4":bool, "Y"=→"7-L_Y_L4":bool, "G"=→"7-L_G_L4":bool)
        n627 = call "Level.vi"("Y_Lev_max"=w951, "IN"=w956, "G_Lev_max"=w953) -> ("R"=→"7-R_R_L4":bool, "Y"=→"7-R_Y_L4":bool, "G"=→"7-R_G_L4":bool)
        n628 = call "Level.vi"("Y_Lev_max"=w951, "IN"=w955, "G_Lev_max"=w953) -> ("R"=→"8-L_R_L4":bool, "Y"=→"8-L_Y_L4":bool, "G"=→"8-L_G_L4":bool)
        n629 = call "Level.vi"("Y_Lev_max"=w951, "IN"=w954, "G_Lev_max"=w953) -> ("R"=→"8-R_R_L4":bool, "Y"=→"8-R_Y_L4":bool, "G"=→"8-R_G_L4":bool)
        n630 = call "Level.vi"("Y_Lev_max"=w343, "IN"=w335, "G_Lev_max"=w341) -> ("R"=→"6-L_R_L4 2":bool, "Y"=→"6-L_Y_L4 2":bool, "G"=→"6-L_G_L4 2":bool)
        n631 = call "Level.vi"("Y_Lev_max"=w343, "IN"=w336, "G_Lev_max"=w341) -> ("R"=→"6-R_R_L4 2":bool, "Y"=→"6-R_Y_L4 2":bool, "G"=→"6-R_G_L4 2":bool)
        n632 = call "Level.vi"("Y_Lev_max"=w343, "IN"=w337, "G_Lev_max"=w341) -> ("R"=→"7-L_R_L4 2":bool, "Y"=→"7-L_Y_L4 2":bool, "G"=→"7-L_G_L4 2":bool)
        n633 = call "Level.vi"("Y_Lev_max"=w343, "IN"=w338, "G_Lev_max"=w341) -> ("R"=→"7-R_R_L4 2":bool, "Y"=→"7-R_Y_L4 2":bool, "G"=→"7-R_G_L4 2":bool)
        n634 = call "Level.vi"("Y_Lev_max"=w343, "IN"=w339, "G_Lev_max"=w341) -> ("R"=→"8-L_R_L4 2":bool, "Y"=→"8-L_Y_L4 2":bool, "G"=→"8-L_G_L4 2":bool)
        n635 = call "Level.vi"("Y_Lev_max"=w343, "IN"=w340, "G_Lev_max"=w341) -> ("R"=→"8-R_R_L4 2":bool, "Y"=→"8-R_Y_L4 2":bool, "G"=→"8-R_G_L4 2":bool)
        n636 = Boolean To (0,1)(Boolean="Logarithm scale 5") -> (0, 1=w1116:i16)
        n637 = Boolean To (0,1)(Boolean="Logarithm scale") -> (0, 1=w1123:i16)
        n638 = Boolean To (0,1)(Boolean="Logarithm scale 3") -> (0, 1=w1120:i16)
        n639 = Boolean To (0,1)(Boolean="Logarithm scale 4") -> (0, 1=w1118:i16)
        n640 = property on="L1 (St-2) -I" class="XYGraph (strict)"("YScale.Mapping Mode"=w1123) -> ()  [unwired: 2 in, 2 out]
        n641 = property on="L2 (St-1) -I" class="XYGraph (strict)"("YScale.Mapping Mode"=w1120) -> ()  [unwired: 2 in, 2 out]
        n642 = property on="L3 (Eta-2) -I" class="XYGraph (strict)"("YScale.Mapping Mode"=w1118) -> ()  [unwired: 2 in, 2 out]
        n643 = property on="L4 (Eta-1) -I" class="XYGraph (strict)"("YScale.Mapping Mode"=w1116) -> ()  [unwired: 2 in, 2 out]
        n644 = Not(x=w1061) -> (.not. x?=→"8-R_Gr_L4":bool)
        n645 = Not(x=w1056) -> (.not. x?=→"8-L_Gr_L4":bool)
        n646 = Not(x=w1060) -> (.not. x?=→"7-R_Gr_L4":bool)
        n647 = Not(x=w1057) -> (.not. x?=→"7-L_Gr_L4":bool)
        n648 = Not(x=w1058) -> (.not. x?=→"6-R_Gr_L4":bool)
        n649 = Not(x=w1059) -> (.not. x?=→"6-L_Gr_L4":bool)
        n650 = Not(x=w311) -> (.not. x?=→"8-R_Gr_L4 2":bool)
        n651 = Not(x=w316) -> (.not. x?=→"8-L_Gr_L4 2":bool)
        n652 = Not(x=w312) -> (.not. x?=→"7-R_Gr_L4 2":bool)
        n653 = Not(x=w315) -> (.not. x?=→"7-L_Gr_L4 2":bool)
        n654 = Not(x=w314) -> (.not. x?=→"6-R_Gr_L4 2":bool)
        n655 = Not(x=w313) -> (.not. x?=→"6-L_Gr_L4 2":bool)
        n656 = Index Array(array=w456, index (row) #1=0 ("index (row)"), index (col) #1=w644, index (row) #2=1 ("index (row)"), index (col) #2=w644, index (row) #3=2 ("index (row)"), index (col) #3=w644, index (row) #4=3 ("index (row)"), index (col) #4=w644, index (row) #5=4 ("index (row)"), index (col) #5=w644, index (row) #6=5 ("index (row)"), index (col) #6=w644) -> (element #1=→"L1_S8-2R_ind 2":dbl, element #2=→"L1_S8-2L_ind 2":dbl, element #3=→"L1_S7-2R_ind 2":dbl, element #4=→"L1_S7-2L_ind 2":dbl, element #5=→"L1_S6-2R_ind 2":dbl, element #6=→"L1_S6-2L_ind 2":dbl)
        n657 = Index Array(array=w454, index (row) #1=0 ("index (row)"), index (col) #1=w620, index (row) #2=1 ("index (row)"), index (col) #2=w620, index (row) #3=2 ("index (row)"), index (col) #3=w620, index (row) #4=3 ("index (row)"), index (col) #4=w620, index (row) #5=4 ("index (row)"), index (col) #5=w620, index (row) #6=5 ("index (row)"), index (col) #6=w620) -> (element #1=→"L3_E8-2R_ind 2":dbl, element #2=→"L3_E8-2L_ind 2":dbl, element #3=→"L3_E7-2R_ind 2":dbl, element #4=→"L3_E7-2L_ind 2":dbl, element #5=→"L3_E6-2R_ind 2":dbl, element #6=→"L3_E6-2L_ind 2":dbl)
        n658 = Index Array(array=w454, index (row) #1=0 ("index (row)"), index (col) #1=w544, index (row) #2=1 ("index (row)"), index (col) #2=w544, index (row) #3=2 ("index (row)"), index (col) #3=w544, index (row) #4=3 ("index (row)"), index (col) #4=w544, index (row) #5=4 ("index (row)"), index (col) #5=w544, index (row) #6=5 ("index (row)"), index (col) #6=w544, index (row) #7=0 ("index (row)"), index (col) #7=w538, index (row) #8=1 ("index (row)"), index (col) #8=w538, index (row) #9=2 ("index (row)"), index (col) #9=w538, index (row) #10=3 ("index (row)"), index (col) #10=w538, index (row) #11=4 ("index (row)"), index (col) #11=w538, index (row) #12=5 ("index (row)"), index (col) #12=w538) -> (element #1=→"E8-2R I 2":dbl, element #2=→"E8-2L I 2":dbl, element #3=→"E7-2R I 2":dbl, element #4=→"E7-2L I 2":dbl, element #5=→"E6-2R I 2":dbl, element #6=→"E6-2L I 2":dbl, element #7=→"E8-2R V 2":dbl, element #8=→"E8-2L V 2":dbl, element #9=→"E7-2R V 2":dbl, element #10=→"E7-2L V 2":dbl, element #11=→"E6-2R V 2":dbl, element #12=→"E6-2L V 2":dbl)
        n659 = Index Array(array=w453, index (row) #1=0 ("index (row)"), index (col) #1=w549, index (row) #2=1 ("index (row)"), index (col) #2=w549, index (row) #3=2 ("index (row)"), index (col) #3=w549, index (row) #4=3 ("index (row)"), index (col) #4=w549, index (row) #5=4 ("index (row)"), index (col) #5=w549, index (row) #6=5 ("index (row)"), index (col) #6=w549, index (row) #7=0 ("index (row)"), index (col) #7=w555, index (row) #8=1 ("index (row)"), index (col) #8=w555, index (row) #9=2 ("index (row)"), index (col) #9=w555, index (row) #10=3 ("index (row)"), index (col) #10=w555, index (row) #11=4 ("index (row)"), index (col) #11=w555, index (row) #12=5 ("index (row)"), index (col) #12=w555) -> (element #1=→"E8-1R I 2":dbl, element #2=→"E8-1L I 2":dbl, element #3=→"E7-1R I 2":dbl, element #4=→"E7-1L I 2":dbl, element #5=→"E6-1R I 2":dbl, element #6=→"E6-1L I 2":dbl, element #7=→"E8-1R V 2":dbl, element #8=→"E8-1L V 2":dbl, element #9=→"E7-1R V 2":dbl, element #10=→"E7-1L V 2":dbl, element #11=→"E6-1R V 2":dbl, element #12=→"E6-1L V 2":dbl)
        n660 = property on="L1 (St-2)  2" class="XYGraph (strict)"("BG Color"="Graphs bachground Color") -> ()  [unwired: 2 in, 2 out]
        n661 = property on="L2 (St-1) 2" class="XYGraph (strict)"("BG Color"="Graphs bachground Color") -> ()  [unwired: 2 in, 2 out]
        n662 = property on="L1 (St-2)" class="XYGraph (strict)"("BG Color"="Graphs bachground Color") -> ()  [unwired: 2 in, 2 out]
        n663 = property on="L2 (St-1)" class="XYGraph (strict)"("BG Color"="Graphs bachground Color") -> ()  [unwired: 2 in, 2 out]
        n664 = property on="Temperature Graph" class="XYGraph (strict)"("BG Color"="Graphs bachground Color") -> ()  [unwired: 2 in, 2 out]
        n665 = property on="Presure Graph" class="XYGraph (strict)"("BG Color"="Graphs bachground Color") -> ()  [unwired: 2 in, 2 out]
        n666 = property on="L3 (Eta-2 )" class="XYGraph (strict)"("BG Color"="Graphs bachground Color") -> ()  [unwired: 2 in, 2 out]
        n667 = property on="L4 (Eta-1)" class="XYGraph (strict)"("BG Color"="Graphs bachground Color") -> ()  [unwired: 2 in, 2 out]
        n668 = Boolean To (0,1)(Boolean="Logarithm scale 10") -> (0, 1=w656:i16)
        n669 = Boolean To (0,1)(Boolean="Logarithm scale 9") -> (0, 1=w657:i16)
        n670 = Boolean To (0,1)(Boolean="Logarithm scale 7") -> (0, 1=w660:i16)
        n671 = Boolean To (0,1)(Boolean="Logarithm scale 8") -> (0, 1=w658:i16)
        n672 = Index Array(array=w1145, index (row) #1=0 ("index (row)"), index (col) #1=w1306, index (row) #2=1 ("index (row)"), index (col) #2=w1306, index (row) #3=2 ("index (row)"), index (col) #3=w1306, index (row) #4=3 ("index (row)"), index (col) #4=w1306, index (row) #5=4 ("index (row)"), index (col) #5=w1306, index (row) #6=5 ("index (row)"), index (col) #6=w1306, index (row) #7=0 ("index (row)"), index (col) #7=w1312, index (row) #8=1 ("index (row)"), index (col) #8=w1312, index (row) #9=2 ("index (row)"), index (col) #9=w1312, index (row) #10=3 ("index (row)"), index (col) #10=w1312, index (row) #11=4 ("index (row)"), index (col) #11=w1312, index (row) #12=5 ("index (row)"), index (col) #12=w1312) -> (element #1=→"E8-2R I":dbl, element #2=→"E8-2L I":dbl, element #3=→"E7-2R I":dbl, element #4=→"E7-2L I":dbl, element #5=→"E6-2R I":dbl, element #6=→"E6-2L I":dbl, element #7=→"E8-2R V":dbl, element #8=→"E8-2L V":dbl, element #9=→"E7-2R V":dbl, element #10=→"E7-2L V":dbl, element #11=→"E6-2R V":dbl, element #12=→"E6-2L V":dbl)
        n673 = Index Array(array=w1144, index (row) #1=0 ("index (row)"), index (col) #1=w1301, index (row) #2=1 ("index (row)"), index (col) #2=w1301, index (row) #3=2 ("index (row)"), index (col) #3=w1301, index (row) #4=3 ("index (row)"), index (col) #4=w1301, index (row) #5=4 ("index (row)"), index (col) #5=w1301, index (row) #6=5 ("index (row)"), index (col) #6=w1301, index (row) #7=0 ("index (row)"), index (col) #7=w1295, index (row) #8=1 ("index (row)"), index (col) #8=w1295, index (row) #9=2 ("index (row)"), index (col) #9=w1295, index (row) #10=3 ("index (row)"), index (col) #10=w1295, index (row) #11=4 ("index (row)"), index (col) #11=w1295, index (row) #12=5 ("index (row)"), index (col) #12=w1295) -> (element #1=→"E8-1R I":dbl, element #2=→"E8-1L I":dbl, element #3=→"E7-1R I":dbl, element #4=→"E7-1L I":dbl, element #5=→"E6-1R I":dbl, element #6=→"E6-1L I":dbl, element #7=→"E8-1R V":dbl, element #8=→"E8-1L V":dbl, element #9=→"E7-1R V":dbl, element #10=→"E7-1L V":dbl, element #11=→"E6-1R V":dbl, element #12=→"E6-1L V":dbl)
        n674 = property on="L1 (St-2) -I 2" class="XYGraph (strict)"("YScale.Mapping Mode"=w660) -> ()  [unwired: 2 in, 2 out]
        n675 = property on="L2 (St-1) -I 2" class="XYGraph (strict)"("YScale.Mapping Mode"=w658) -> ()  [unwired: 2 in, 2 out]
        n676 = property on="L3 (Eta-2) -I 2" class="XYGraph (strict)"("YScale.Mapping Mode"=w657) -> ()  [unwired: 2 in, 2 out]
        n677 = property on="L4 (Eta-1) -I 2" class="XYGraph (strict)"("YScale.Mapping Mode"=w656) -> ()  [unwired: 2 in, 2 out]
        n678 = property on="L3 (Eta-2 ) 2" class="XYGraph (strict)"("BG Color"="Graphs bachground Color") -> ()  [unwired: 2 in, 2 out]
        n679 = property on="L4 (Eta-1) 2" class="XYGraph (strict)"("BG Color"="Graphs bachground Color") -> ()  [unwired: 2 in, 2 out]
      }
      n680 = call <instrlib>:"CAENHV Deinit System.vi"("error in (no error)"=w160, "handle"=w159) -> ()  [unwired: 9 in, 1 out]
    }
  }
